vi "数据采集传输系统.vi"() -> ()   [LabVIEW 2016]
uses:
  <vilib>/Utility/miscctls.llb/LVPointTypeDef.ctl
  <vilib>/Utility/config.llb/Write Key (String).vi
  <vilib>/Utility/config.llb/Read Key (String).vi
  <vilib>/Utility/config.llb/Read Key (Boolean).vi
  <vilib>/Utility/config.llb/Read Key (I32).vi
  <vilib>/Utility/config.llb/Write Key (U32).vi
  <vilib>/Utility/config.llb/Write Key (Boolean).vi
  <vilib>/Utility/config.llb/Write Key (I32).vi
  <vilib>/Utility/config.llb/NI_LVConfig.lvlib
  data/FreeMem.dll
  <vilib>/ptbypt/NI_PtbyPt.lvlib
panel:
  in  "数组大小":i32
  in  "实时数据发送时间间隔/min":i32=1
  in  "数据组合发送":bool
  in  "日志、参数发送":bool
  in  "2011发送":bool
  in  "判断数据反馈":bool
  in  "数据发送协议":enum16{"2005-212协议", "2017-212协议"}(ring)=enum."2017-212协议"
  in  "数据发送通道":enum16{"TCP", "VISA"}(ring)
  in  "baud rate":u32=9600 caption="波特率"
  in  "VISA resource name":refnum<visa-resource-name> caption="VISA资源名称"
  in  "查询质控数据起始时间":bool
  in  "返回主界面":bool
  out "零点核查索引起始时间":string
  out "跨度核查索引起始时间":string
  out "加标回收索引起始时间":string
  out "标样核查索引起始时间":string
  out "数据接收超时指示灯":bool
  in  "重发时间":T1(ring)
  in  "重发日期":T2(ring)
  in  "锁":bool
  in  "开机启动":bool
  in  "确定更改起始时间":bool
  in  "更改起始时间":bool
  in  "数据发送起始时间":timestamp format="%<%.3X\n%Y/%m/%d>T"
  in  "每周自动重发":bool=TRUE
  in  "确定":bool
  in  "返回":bool
  in  "PW":string
  in  "MN":string
  in  "PORT":string
  in  "IP":string
  in  "站点设备":string
  in  "站点名称":string
  out "设置超时时间/min":i32=1
  out "空闲时间/s":string
  out "状态信息":T3={"1st Error to Convert "=63, "步骤 "=enum."打开连接", "元素"="实时数据", "TCP服务端掉线计数"=4, "TCP掉线时间节点"="2019/05/08 15:24:17"} {"1st Error to Convert" items=["无错误", "参数错误", "内存已满", "超出区域", "文件结束", "文件已打开", "一般文件IO错误", "未找到文件", "文件权限错误", "磁盘已满", "路径副本", "打开过多文件", "未启用", "未找到资源文件", "无法添加资源", "未找到资源", "未找到图像", "图像内存错误", "画笔不存在", "配置错误类型", "配置未找到解析段", "配置解析错误", "配置内存错误", "错误外部代码格式", "错误外部代码偏移量", "外部代码不存在", "空窗口", "销毁窗口错误", "空菜单", "打印已中止", "错误打印记录", "打印驱动程序错误", "打印时窗口错误", "打印时内存错误", "打印对话框错误", "一般打印错误", "无效设备引用句柄", "设备未找到", "设备参数错误", "设备单位错误", "无法打开设备", "设备调用已中止", "一般错误", "用户已取消", "对象ID过低", "对象ID过高", "对象不在堆中", "未知的堆", "错误DefProc ID", "DefProc不在表格中", "范围外信息", "空方法", "未知信息", "不支持管理器调用", "错误地址", "连接过程中", "连接超时", "连接过程中", "不支持网络属性", "网络错误", "正在使用的地址", "系统缺少内存", "连接已中止", "连接已拒绝", "连接未建立", "连接已建立", "连接已关闭", "初始化错误（交互应用程序管理器）", "错误事件发生", "等待无约束事件发生处理程序", "事件发生队列溢出", "错误路径", "未发出信号量", "未识别类型（交互应用程序管理器）"]}
  out "系统时间":string
  out "实时小时数据上传":bool
  out "系统状态改变":bool
  out "软件版本":string
  out "掉线指示":bool
  out "核查数据上传":bool
  out "通信状态":bool
  out "配置信息":T4
  in  "参数配置":bool
  out "查询数据发送":bool
  out "读取报文显示":string
  out "发送报文显示":string
  out "心跳包":bool
  in  "参数数值":T5={"CODMn"=TRUE, "CODCr"=TRUE, "DO"=TRUE, "铜"=TRUE, "PH"=TRUE, "氨氮"=TRUE, "比电导率"=TRUE, "水温"=TRUE, "盐度(海水)"=TRUE, "浊度"=TRUE, "总氮"=TRUE, "总磷"=TRUE, "叶绿素a"=TRUE, "藻密度"=TRUE, "水位"=TRUE, "流速"=TRUE, "瞬时流量"=TRUE, "累积流量"=TRUE}
  in  "系统编码选择框":string(combo)="地表水质量监测"
  out "主队列输出":refnum<queue>
  in  "TCP掉线时间节点":string
  out "TCP服务端掉线计数":i32
  out "元素":string
  out "步骤":T6(ring)
  out "1st Error to Convert":i32(ring)=56 items=["无错误", "参数错误", "内存已满", "超出区域", "文件结束", "文件已打开", "一般文件IO错误", "未找到文件", "文件权限错误", "磁盘已满", "路径副本", "打开过多文件", "未启用", "未找到资源文件", "无法添加资源", "未找到资源", "未找到图像", "图像内存错误", "画笔不存在", "配置错误类型", "配置未找到解析段", "配置解析错误", "配置内存错误", "错误外部代码格式", "错误外部代码偏移量", "外部代码不存在", "空窗口", "销毁窗口错误", "空菜单", "打印已中止", "错误打印记录", "打印驱动程序错误", "打印时窗口错误", "打印时内存错误", "打印对话框错误", "一般打印错误", "无效设备引用句柄", "设备未找到", "设备参数错误", "设备单位错误", "无法打开设备", "设备调用已中止", "一般错误", "用户已取消", "对象ID过低", "对象ID过高", "对象不在堆中", "未知的堆", "错误DefProc ID", "DefProc不在表格中", "范围外信息", "空方法", "未知信息", "不支持管理器调用", "错误地址", "连接过程中", "连接超时", "连接过程中", "不支持网络属性", "网络错误", "正在使用的地址", "系统缺少内存", "连接已中止", "连接已拒绝", "连接未建立", "连接已建立", "连接已关闭", "初始化错误（交互应用程序管理器）", "错误事件发生", "等待无约束事件发生处理程序", "事件发生队列溢出", "错误路径", "未发出信号量", "未识别类型（交互应用程序管理器）"]
  out "QN":string
  out "时间QN":string
  out "系统编码ST":string
  out "命令编码CN":string
  out "密码PW":string
  out "设备编码MN":string
  out "拆分包及应答Flag":string
  out "数据":string
  in  "实时数据参数选择框":T7={"水样测量数据"=FALSE, "零点核查数据"=TRUE, "跨度核查数据"=TRUE, "加标回收数据"=TRUE, "平行样数据"=FALSE, "标样核查"=TRUE, "集成干预测试"=TRUE}
  out "数据输出":string
  in  "table元素":string
  out "空闲时间":dbl
  # "数 据 采 集 传 输 系 统"
  # "读取的参数区"
  # "水样测量数据"
  # "空白测试数据"
  # "跨度核查数据"
  # "加标回收数据"
  # "平行样数据"
  # "标样核查"
  # "集成干预测试"
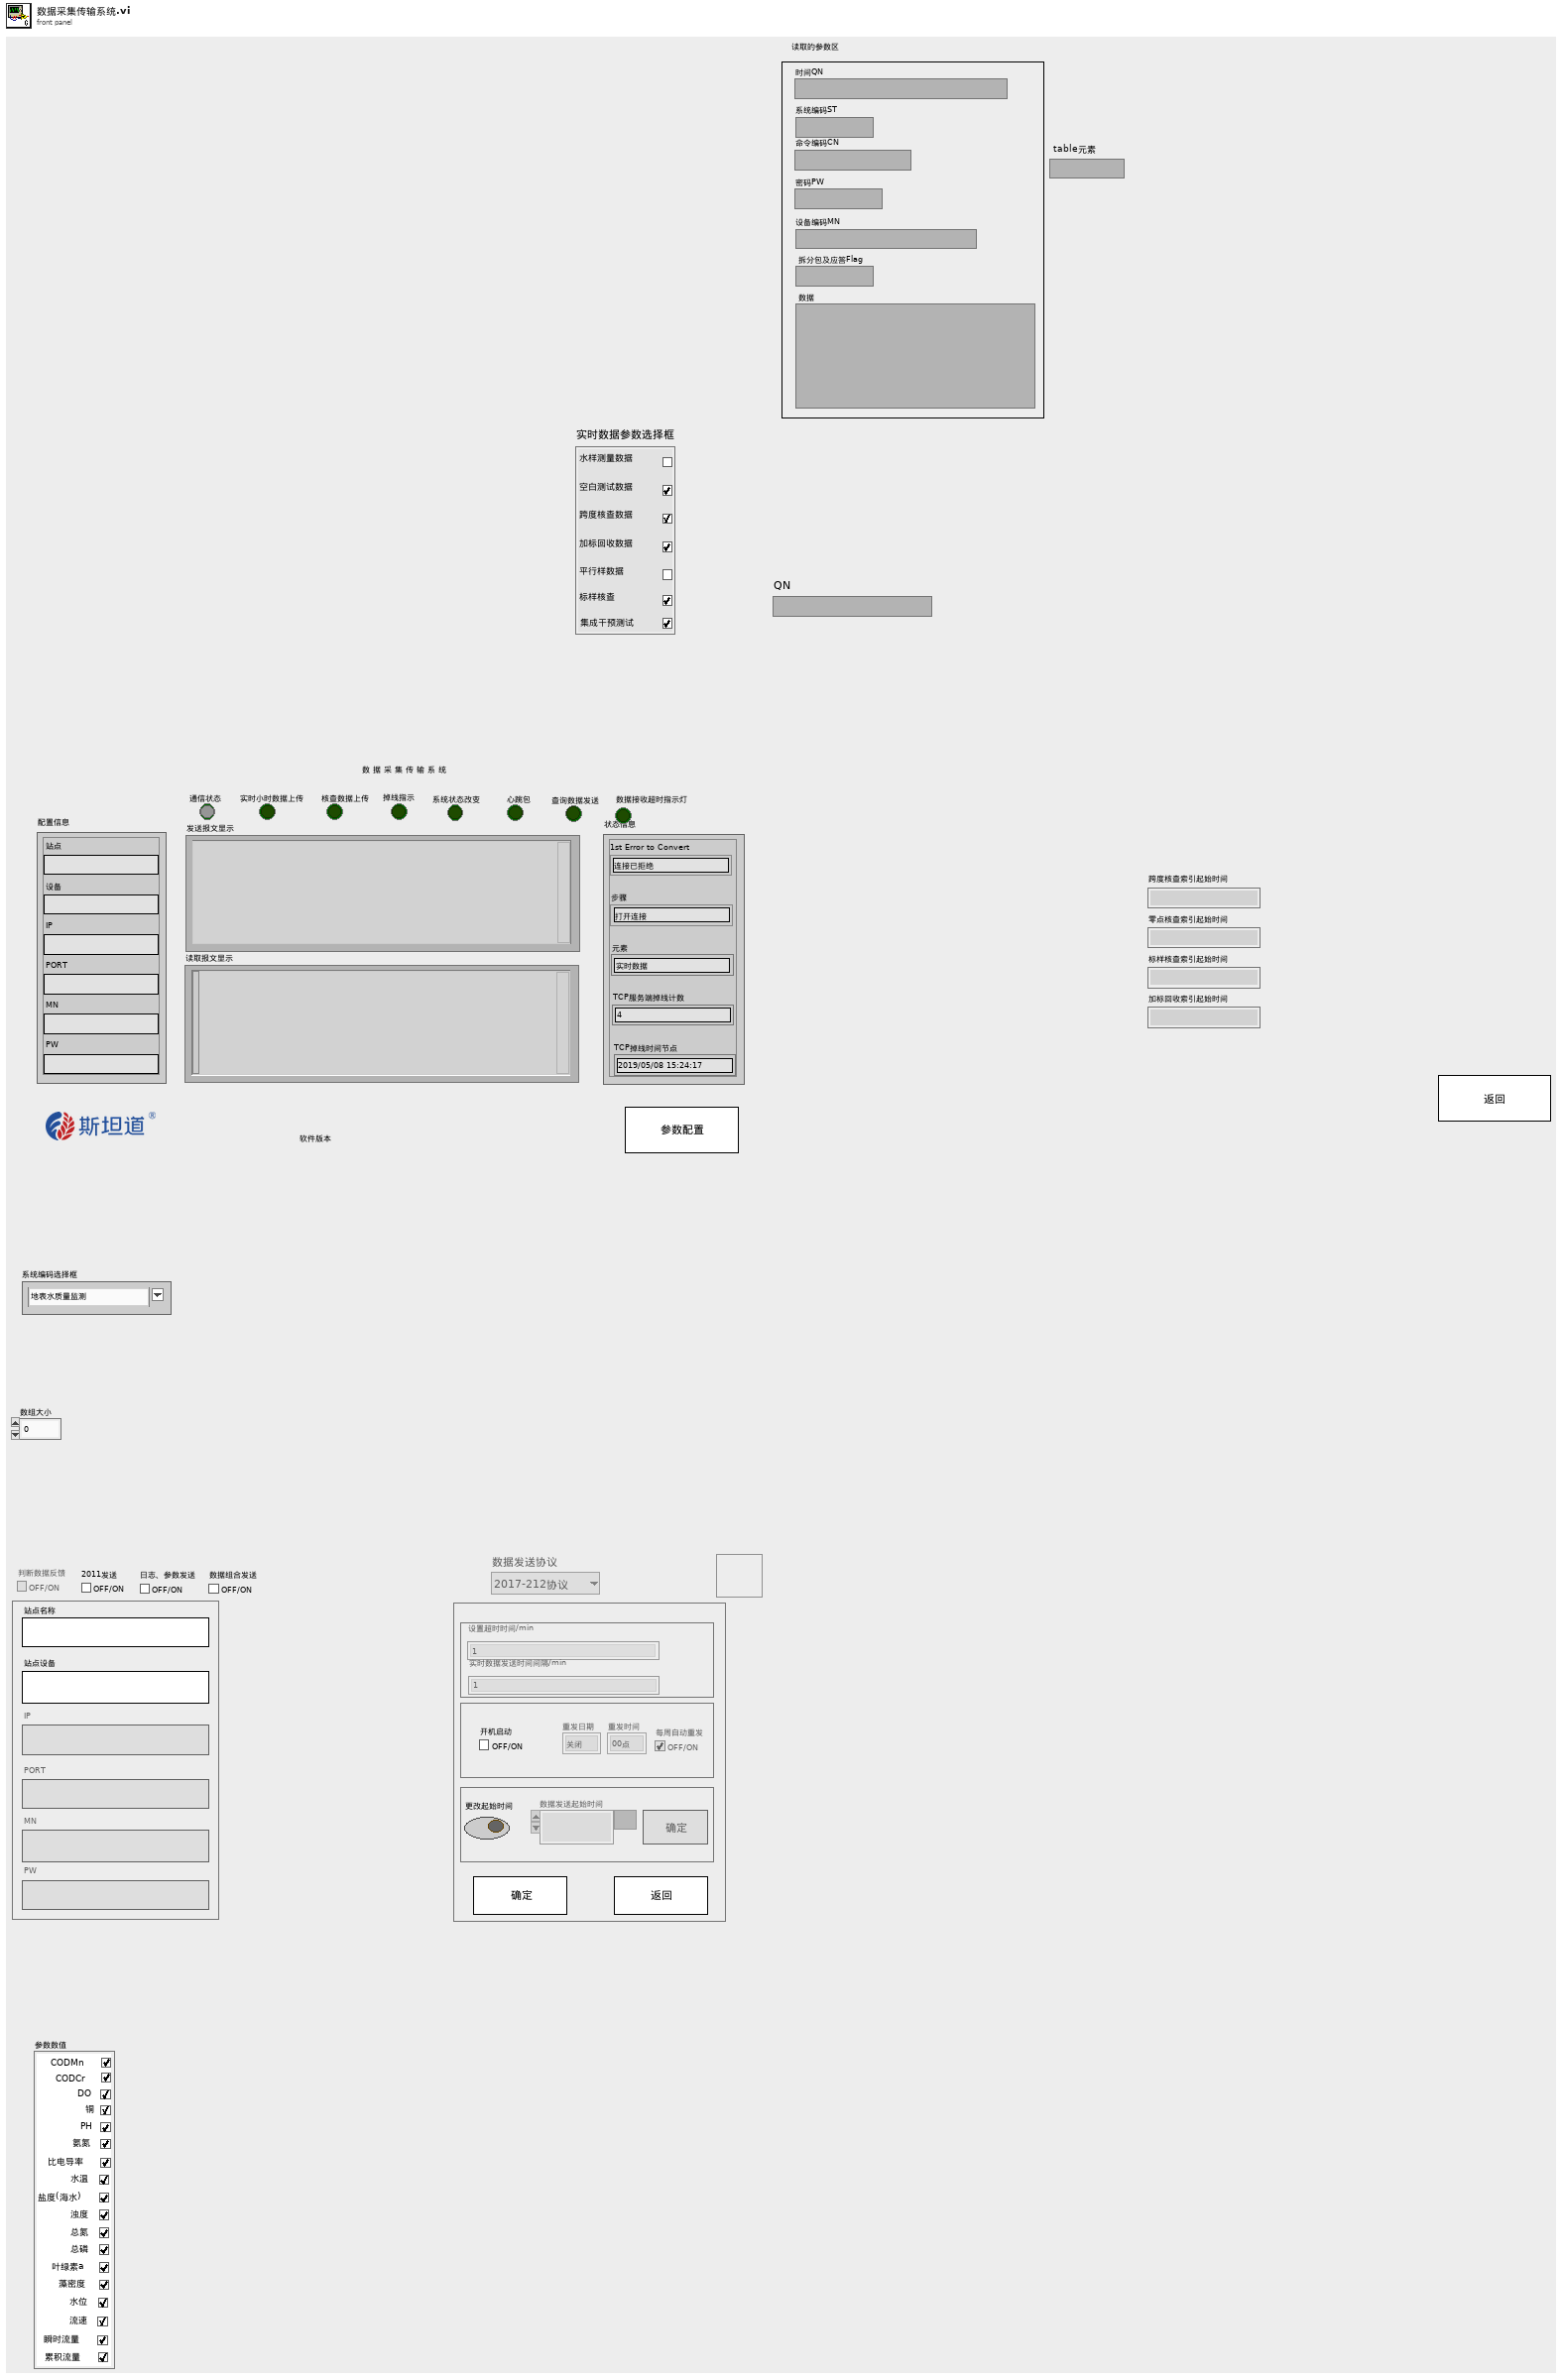
[diagram p1: front panel]
types:
  T1 = enum16{"00点", "01点", "02点", "03点", "04点", "05点", "06点", "07点", "08点", "09点", "10点", "11点", "12点", "13点", "14点", "15点", "16点", "17点", "18点", "19点", "20点", "21点", "22点", "23点"}
  T2 = enum16{"关闭", "星期日", "星期一", "星期二", "星期三", "星期四", "星期五", "星期六"}
  T3 = cluster{"1st Error to Convert ":i32, "步骤 ":enum16{"初始化", "打开连接", "表格比对", "发送数据", "读取数据", "数据处理"}, "元素":string, "TCP服务端掉线计数":i32, "TCP掉线时间节点":string}
  T4 = cluster{"站点":string, "设备":string, "IP":string, "PORT":string, "MN":string, "PW":string}
  T5 = cluster{"CODMn":bool, "CODCr":bool, "DO":bool, "铜":bool, "PH":bool, "氨氮":bool, "比电导率":bool, "水温":bool, "盐度(海水)":bool, "浊度":bool, "总氮":bool, "总磷":bool, "叶绿素a":bool, "藻密度":bool, "水位":bool, "流速":bool, "瞬时流量":bool, "累积流量":bool}
  T6 = enum16{"初始化", "打开连接", "表格比对", "发送数据", "读取数据", "数据处理"}
  T7 = cluster{"水样测量数据":bool, "零点核查数据":bool, "跨度核查数据":bool, "加标回收数据":bool, "平行样数据":bool, "标样核查":bool, "集成干预测试":bool}
  T8 = typedef "NI_LVConfig.lvlib/Config Data RefNum.ctl" = refnum<k1>
  T9 = typedef "LVDateTimeRec.ctl" = cluster{"秒数的小数部分":dbl, "秒":i32, "分":i32, "时":i32, "日":i32, "月":i32, "年":i32, "天数（周）":i32, "天数（年）":i32, "DST":i32}
  T10 = enum8{"Enabled", "Disabled", "Disabled and Grayed Out"}
  T11 = typedef "LVPointTypeDef.ctl" = cluster{"Horizontal":i16, "Vertical":i16}
  T12 = enum16{"水样测试", "小时数据", "日志信息", "报警信息", "零点核查", "标样核查", "平行样", "加标回收"}
  T13 = typedef "imagedata.ctl" = cluster{"image type":i32, "image depth":i32, "image":u8[], "mask":u8[], "colors":u32[], "Rectangle":cluster{"left":i16, "top":i16, "right":i16, "bottom":i16}}
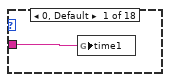
[diagram p5: hidden frame]
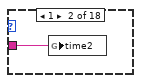
[diagram p6: hidden frame]
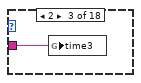
[diagram p7: hidden frame]
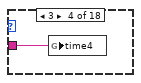
[diagram p8: hidden frame]
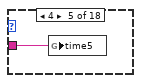
[diagram p9: hidden frame]
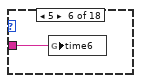
[diagram p10: hidden frame]
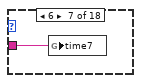
[diagram p11: hidden frame]
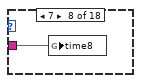
[diagram p12: hidden frame]
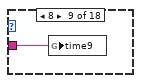
[diagram p13: hidden frame]
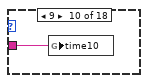
[diagram p14: hidden frame]
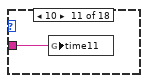
[diagram p15: hidden frame]
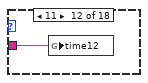
[diagram p16: hidden frame]
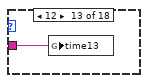
[diagram p17: hidden frame]
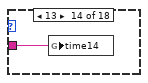
[diagram p18: hidden frame]
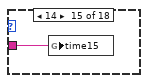
[diagram p19: hidden frame]
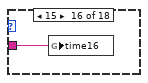
[diagram p20: hidden frame]
diagram:
  w37 = 0 ("索引")
  # "上传本地时间点的实时数据"
  # "目前时间太短，如果掉线了，数据存不了临时表格"
  n1 = Cluster To Array(cluster="参数数值") -> (array=w47:bool[])
  n2 = for {
    tunnel: w47 -> [_] mode=indexing
    tunnel: [w73] -> _
    i -> [w73]
    w62 = "线程一数据重发功能" ("section")
    # "初始化水样搜索起始时间"
    n3 = case shown="3" w73 {
      tunnel: [w104 w106 w108 w110 w112 w114 w116 w118 w120 w122 w124 w126 w128 w130 w132 w134 w136 w138] -> w77
      frame 0, Default {
        n4 = control-ref of="CODMn"() -> (w105:refnum<vi>)
        n5 = property class="Bool (严格)"(reference=w105) -> ("Label.Text"=w104:string)  [unwired: 1 in, 2 out]
      }
      frame 1 {
        n6 = control-ref of="CODCr"() -> (w107:refnum<vi>)
        n7 = property class="Bool (严格)"(reference=w107) -> ("Label.Text"=w106:string)  [unwired: 1 in, 2 out]
      }
      frame 2 {
        n8 = control-ref of="DO"() -> (w109:refnum<vi>)
        n9 = property class="Bool (严格)"(reference=w109) -> ("Label.Text"=w108:string)  [unwired: 1 in, 2 out]
      }
      frame 3 {
        n10 = control-ref of="铜"() -> (w111:refnum<vi>)
        n11 = property class="Bool (严格)"(reference=w111) -> ("Label.Text"=w110:string)  [unwired: 1 in, 2 out]
      }
      frame 4 {
        n12 = control-ref of="PH"() -> (w113:refnum<vi>)
        n13 = property class="Bool (严格)"(reference=w113) -> ("Label.Text"=w112:string)  [unwired: 1 in, 2 out]
      }
      frame 5 {
        n14 = control-ref of="氨氮"() -> (w115:refnum<vi>)
        n15 = property class="Bool (严格)"(reference=w115) -> ("Label.Text"=w114:string)  [unwired: 1 in, 2 out]
      }
      frame 6 {
        n16 = control-ref of="比电导率"() -> (w117:refnum<vi>)
        n17 = property class="Bool (严格)"(reference=w117) -> ("Label.Text"=w116:string)  [unwired: 1 in, 2 out]
      }
      frame 7 {
        n18 = control-ref of="水温"() -> (w119:refnum<vi>)
        n19 = property class="Bool (严格)"(reference=w119) -> ("Label.Text"=w118:string)  [unwired: 1 in, 2 out]
      }
      frame 8 {
        n20 = control-ref of="盐度(海水)"() -> (w121:refnum<vi>)
        n21 = property class="Bool (严格)"(reference=w121) -> ("Label.Text"=w120:string)  [unwired: 1 in, 2 out]
      }
      frame 9 {
        n22 = control-ref of="浊度"() -> (w123:refnum<vi>)
        n23 = property class="Bool (严格)"(reference=w123) -> ("Label.Text"=w122:string)  [unwired: 1 in, 2 out]
      }
      frame 10 {
        n24 = control-ref of="总氮"() -> (w125:refnum<vi>)
        n25 = property class="Bool (严格)"(reference=w125) -> ("Label.Text"=w124:string)  [unwired: 1 in, 2 out]
      }
      frame 11 {
        n26 = control-ref of="总磷"() -> (w127:refnum<vi>)
        n27 = property class="Bool (严格)"(reference=w127) -> ("Label.Text"=w126:string)  [unwired: 1 in, 2 out]
      }
      frame 12 {
        n28 = control-ref of="叶绿素a"() -> (w129:refnum<vi>)
        n29 = property class="Bool (严格)"(reference=w129) -> ("Label.Text"=w128:string)  [unwired: 1 in, 2 out]
      }
      frame 13 {
        n30 = control-ref of="藻密度"() -> (w131:refnum<vi>)
        n31 = property class="Bool (严格)"(reference=w131) -> ("Label.Text"=w130:string)  [unwired: 1 in, 2 out]
      }
      frame 14 {
        n32 = control-ref of="水位"() -> (w133:refnum<vi>)
        n33 = property class="Bool (严格)"(reference=w133) -> ("Label.Text"=w132:string)  [unwired: 1 in, 2 out]
      }
      frame 15 {
        n34 = control-ref of="流速"() -> (w135:refnum<vi>)
        n35 = property class="Bool (严格)"(reference=w135) -> ("Label.Text"=w134:string)  [unwired: 1 in, 2 out]
      }
      frame 16 {
        n36 = control-ref of="瞬时流量"() -> (w137:refnum<vi>)
        n37 = property class="Bool (严格)"(reference=w137) -> ("Label.Text"=w136:string)  [unwired: 1 in, 2 out]
      }
      frame 17 {
        n38 = control-ref of="累积流量"() -> (w139:refnum<vi>)
        n39 = property class="Bool (严格)"(reference=w139) -> ("Label.Text"=w138:string)  [unwired: 1 in, 2 out]
      }
    }
    n40 = call <vilib>:"Application Directory.vi"() -> ("Application Directory"=w83:path)
    n41 = Build Path(base path=w83, name or relative path="data\\Set.ini" ("名称或相对路径")) -> (appended path=w81:path)
    n42 = call <vilib>:"Open Config Data.vi"("configuration file path"=w81) -> ("error out"=w79:errorcluster, "refnum"=w80:T8)  [unwired: 8 in, 1 out]
    n43 = call-poly <vilib>:"Read Key.vi"("section"="线程一数据搜索起始时间", "error in (no error)"=w79, "key"=w77, "refnum"=w80) -> ("error out"=w71:errorcluster, "value"=w74:string, "refnum out"=w72:T8)  [unwired: 4 in, 1 out]
    n44 = Empty String/Path?(string/path=w74) -> (empty?=w76:bool)
    n45 = case shown="真" w76 {
      tunnel: [w84 "1904/01/01 00:00:00"] -> w75
      tunnel: w74 -> [w84 _]
      frame False {
      }
      frame True {
      }
    }
    n46 = call-poly <vilib>:"Read Key.vi"("section"=w62, "error in (no error)"=w71, "key"="重发功能", "refnum"=w72) -> ("error out"=w65:errorcluster, "value"=w69:bool, "refnum out"=w66:T8)  [unwired: 4 in, 1 out]
    n47 = local write "每周自动重发"(w69) -> ()
    n48 = call-poly <vilib>:"Read Key.vi"("section"=w62, "error in (no error)"=w65, "key"="重发日期", "refnum"=w66) -> ("error out"=w63:errorcluster, "value"=w59:i32, "refnum out"=w64:T8)  [unwired: 4 in, 1 out]
    n49 = local write "重发日期"(w59) -> ()
    n50 = case shown="3" w73 {
      tunnel: w75 -> [w86 w87 w88 w89 w90 w91 w92 w93 w94 w95 w96 w97 w98 w99 w100 w101 w102 w103]
      frame 0, Default {
        n51 = global write "全局 水样时间.vi" "time1"(w86) -> ()
      }
      frame 1 {
        n52 = global write "全局 水样时间.vi" "time2"(w87) -> ()
      }
      frame 2 {
        n53 = global write "全局 水样时间.vi" "time3"(w88) -> ()
      }
      frame 3 {
        n54 = global write "全局 水样时间.vi" "time4"(w89) -> ()
      }
      frame 4 {
        n55 = global write "全局 水样时间.vi" "time5"(w90) -> ()
      }
      frame 5 {
        n56 = global write "全局 水样时间.vi" "time6"(w91) -> ()
      }
      frame 6 {
        n57 = global write "全局 水样时间.vi" "time7"(w92) -> ()
      }
      frame 7 {
        n58 = global write "全局 水样时间.vi" "time8"(w93) -> ()
      }
      frame 8 {
        n59 = global write "全局 水样时间.vi" "time9"(w94) -> ()
      }
      frame 9 {
        n60 = global write "全局 水样时间.vi" "time10"(w95) -> ()
      }
      frame 10 {
        n61 = global write "全局 水样时间.vi" "time11"(w96) -> ()
      }
      frame 11 {
        n62 = global write "全局 水样时间.vi" "time12"(w97) -> ()
      }
      frame 12 {
        n63 = global write "全局 水样时间.vi" "time13"(w98) -> ()
      }
      frame 13 {
        n64 = global write "全局 水样时间.vi" "time14"(w99) -> ()
      }
      frame 14 {
        n65 = global write "全局 水样时间.vi" "time15"(w100) -> ()
      }
      frame 15 {
        n66 = global write "全局 水样时间.vi" "time16"(w101) -> ()
      }
      frame 16 {
        n67 = global write "全局 水样时间.vi" "time17"(w102) -> ()
      }
      frame 17 {
        n68 = global write "全局 水样时间.vi" "time18"(w103) -> ()
      }
    }
    n69 = call-poly <vilib>:"Read Key.vi"("section"=w62, "error in (no error)"=w63, "key"="重发时间", "refnum"=w64) -> ("error out"=w60:errorcluster, "value"=w58:i32, "refnum out"=w61:T8)  [unwired: 4 in, 1 out]
    n70 = local write "重发时间"(w58) -> ()
    n71 = call <vilib>:"Close Config Data.vi"("error in (no error)"=w60, "refnum"=w61) -> ()  [unwired: 8 in, 2 out]
  }
  n72 = vi-ref "数据传输系统.lvlib:核查数据和日志信息入发送队列 (子VI).vi"() -> (w20:refnum<vi>)
  n73 = vi-ref "数据传输系统.lvlib:主动上传工控机周期和模式 (子VI).vi"() -> (w29:refnum<vi>)
  n74 = vi-ref "数据传输系统.lvlib:核查数据和日志信息出发送队列 (子VI).vi"() -> (w11:refnum<vi>)
  n75 = local read "实时小时数据上传"() -> (w16:bool)
  n76 = property class="VI"(reference=w29) -> ("Name"=w30:string)  [unwired: 1 in, 2 out]
  n77 = property class="VI"(reference=w11) -> ("Name"=w10:string)  [unwired: 1 in, 2 out]
  n78 = local read "查询数据发送"() -> (w3:bool)
  n79 = local read "核查数据上传"() -> (w19:bool)
  n80 = local read "查询数据发送"() -> (w18:bool)
  n81 = local read "日志、参数发送"() -> (w14:bool)
  n82 = property class="VI"(reference=w20) -> ("Name"=w27:string)  [unwired: 1 in, 2 out]
  n83 = local read "步骤"() -> (w17:T6)
  n84 = local read "数据发送协议"() -> (w15:enum16{"2005-212协议", "2017-212协议"})
  n85 = Open VI Reference(type specifier VI Refnum (for type only)=refnum<vi> refnum, vi path=w30, options=128 ("选项")) -> (vi reference=w32:refnum<vi>, error out=w34:errorcluster)  [unwired: 3 in]
  n86 = Open VI Reference(type specifier VI Refnum (for type only)=refnum<vi> refnum, vi path=w10, options=128 ("选项")) -> (vi reference=w8:refnum<vi>, error out=w6:errorcluster)  [unwired: 3 in]
  n87 = Open VI Reference(type specifier VI Refnum (for type only)=refnum<vi> refnum, vi path=w27, options=128 ("选项")) -> (vi reference=w25:refnum<vi>, error out=w23:errorcluster)  [unwired: 3 in]
  n88 = call-by-ref "?"(reference=w32, error in=w34) -> (reference out=w36:refnum<vi>, error out=w35:errorcluster, "系统状态改变"=→"系统状态改变":bool)  [unwired: 11 in]
  n89 = call-by-ref "?"(reference=w8, error in=w6, "查询数据发送"=w3) -> (reference out=w4:refnum<vi>, error out=w5:errorcluster, "核查数据上传"=→"核查数据上传":bool)  [unwired: 10 in]
  n90 = call-by-ref "?"(reference=w25, error in=w23, "实时数据参数选择框"="实时数据参数选择框", "实时数据发送时间间隔/min"="实时数据发送时间间隔/min", "日志、参数发送输入"=w14, "数据发送协议输入"=w15, "实时小时数据上传输入"=w16, "步骤输入"=w17, "查询数据发送输入"=w18, "核查数据上传输入"=w19) -> (reference out=w21:refnum<vi>, error out=w22:errorcluster)  [unwired: 4 in]
  n91 = Close Reference(reference=w36, error in (no error)=w35) -> ()  [unwired: 1 out]
  n92 = Close Reference(reference=w4, error in (no error)=w5) -> ()  [unwired: 1 out]
  n93 = Close Reference(reference=w21, error in (no error)=w22) -> ()  [unwired: 1 out]
  n94 = while "While循环" {
    tunnel: [w154] -> _
    stop <- FALSE stop-if-true
    w145 = FALSE ("小时数据上传")
    # "2017，2005版协议实时、小时数据出数据就单参数上传"
    n95 = local read "查询数据发送"() -> (w147:bool)
    n96 = local read "核查数据上传"() -> (w146:bool)
    n97 = global read "全局 数据发送重叠.vi" "掉线指示灯"() -> (w141:bool)
    n98 = local read "步骤"() -> (w153:T6)
    n99 = local write "实时小时数据上传"(w145) -> ()
    n100 = global write "全局 数据发送重叠.vi" "主动上报数据中"(w145) -> ()
    n101 = Greater Or Equal?(x="数组大小", y=17) -> (x >= y?=w150:bool)
    n102 = Not(x=w141) -> (.not. x?=w140:bool)
    n103 = Not(x=w147) -> (.not. x?=w144:bool)
    n104 = Not(x=w146) -> (.not. x?=w143:bool)
    n105 = Equal?(x=w153, y=T6."读取数据" ("步骤")) -> (x = y?=w151:bool)
    n106 = Wait (ms)(milliseconds to wait=u32 75430 ("等待时间（毫秒）")) -> ()  [unwired: 1 out]
    n107 = Compound Arithmetic op=AND ("复合运算")(w151, w140, w150, w144, w143) -> (w148:bool)
    n108 = case shown="真" w148 {
      tunnel: [_ w159] -> w154
      frame False {
        w157 = FALSE ("小时数据上传")
        n109 = local write "实时小时数据上传"(w157) -> ()
        n110 = global write "全局 数据发送重叠.vi" "主动上报数据中"(w157) -> ()
      }
      frame True {
        n111 = global read "断电保存全局.vi" "数据组合发送"() -> (w158:bool)
        n112 = case shown="假" w158 {
          tunnel: [w160 _] -> w159
          frame False {
            # "数据非整点触发，而是实时触发，分条发送"
            n113 = flat-sequence {
              tunnel: [w164] -> w161
              tunnel: [w445] -> w160
              tunnel: w161 -> [w445]
              frame #0 {
                w163 = TRUE ("小时数据上传")
                n114 = global read "断电保存全局.vi" "数据发送协议"() -> (w162:enum16{"2005-212协议", "2017-212协议"})
                n115 = global write "全局 数据发送重叠.vi" "主动上报数据中"(w163) -> ()
                n116 = case shown="\"2017-212协议\", 默认" w162 {
                  tunnel: [_ w266] -> w164
                  frame "2005-212协议" {
                    n117 = local read "参数数值"() -> (w165:T5)
                    n118 = Cluster To Array(cluster=w165) -> (array=w168:bool[])
                    n119 = for {
                      tunnel: w168 -> [_] mode=indexing
                      tunnel: [w211] -> w167
                      i -> [w209]
                      (unwired) " where 时间 between #"
                      w207 = "database1.mdb" ("database")
                      (unwired) "'and 数据类型 ='N' and 时间 between "
                      n120 = case shown="12" w209 {
                        tunnel: [w230 w232 w234 w236 w238 w240 w242 w244 w246 w248 w250 w252 w254 w256 w258 w260 w262 w264] -> w208
                        frame 0, Default {
                          n121 = control-ref of="CODMn"() -> (w231:refnum<vi>)
                          n122 = property class="Bool (严格)"(reference=w231) -> ("Label.Text"=w230:string)  [unwired: 1 in, 2 out]
                        }
                        frame 1 {
                          n123 = control-ref of="CODCr"() -> (w233:refnum<vi>)
                          n124 = property class="Bool (严格)"(reference=w233) -> ("Label.Text"=w232:string)  [unwired: 1 in, 2 out]
                        }
                        frame 2 {
                          n125 = control-ref of="DO"() -> (w235:refnum<vi>)
                          n126 = property class="Bool (严格)"(reference=w235) -> ("Label.Text"=w234:string)  [unwired: 1 in, 2 out]
                        }
                        frame 3 {
                          n127 = control-ref of="铜"() -> (w237:refnum<vi>)
                          n128 = property class="Bool (严格)"(reference=w237) -> ("Label.Text"=w236:string)  [unwired: 1 in, 2 out]
                        }
                        frame 4 {
                          n129 = control-ref of="PH"() -> (w239:refnum<vi>)
                          n130 = property class="Bool (严格)"(reference=w239) -> ("Label.Text"=w238:string)  [unwired: 1 in, 2 out]
                        }
                        frame 5 {
                          n131 = control-ref of="氨氮"() -> (w241:refnum<vi>)
                          n132 = property class="Bool (严格)"(reference=w241) -> ("Label.Text"=w240:string)  [unwired: 1 in, 2 out]
                        }
                        frame 6 {
                          n133 = control-ref of="比电导率"() -> (w243:refnum<vi>)
                          n134 = property class="Bool (严格)"(reference=w243) -> ("Label.Text"=w242:string)  [unwired: 1 in, 2 out]
                        }
                        frame 7 {
                          n135 = control-ref of="水温"() -> (w245:refnum<vi>)
                          n136 = property class="Bool (严格)"(reference=w245) -> ("Label.Text"=w244:string)  [unwired: 1 in, 2 out]
                        }
                        frame 8 {
                          n137 = control-ref of="盐度(海水)"() -> (w247:refnum<vi>)
                          n138 = property class="Bool (严格)"(reference=w247) -> ("Label.Text"=w246:string)  [unwired: 1 in, 2 out]
                        }
                        frame 9 {
                          n139 = control-ref of="浊度"() -> (w249:refnum<vi>)
                          n140 = property class="Bool (严格)"(reference=w249) -> ("Label.Text"=w248:string)  [unwired: 1 in, 2 out]
                        }
                        frame 10 {
                          n141 = control-ref of="总氮"() -> (w251:refnum<vi>)
                          n142 = property class="Bool (严格)"(reference=w251) -> ("Label.Text"=w250:string)  [unwired: 1 in, 2 out]
                        }
                        frame 11 {
                          n143 = control-ref of="总磷"() -> (w253:refnum<vi>)
                          n144 = property class="Bool (严格)"(reference=w253) -> ("Label.Text"=w252:string)  [unwired: 1 in, 2 out]
                        }
                        frame 12 {
                          n145 = control-ref of="叶绿素a"() -> (w255:refnum<vi>)
                          n146 = property class="Bool (严格)"(reference=w255) -> ("Label.Text"=w254:string)  [unwired: 1 in, 2 out]
                        }
                        frame 13 {
                          n147 = control-ref of="藻密度"() -> (w257:refnum<vi>)
                          n148 = property class="Bool (严格)"(reference=w257) -> ("Label.Text"=w256:string)  [unwired: 1 in, 2 out]
                        }
                        frame 14 {
                          n149 = control-ref of="水位"() -> (w259:refnum<vi>)
                          n150 = property class="Bool (严格)"(reference=w259) -> ("Label.Text"=w258:string)  [unwired: 1 in, 2 out]
                        }
                        frame 15 {
                          n151 = control-ref of="流速"() -> (w261:refnum<vi>)
                          n152 = property class="Bool (严格)"(reference=w261) -> ("Label.Text"=w260:string)  [unwired: 1 in, 2 out]
                        }
                        frame 16 {
                          n153 = control-ref of="瞬时流量"() -> (w263:refnum<vi>)
                          n154 = property class="Bool (严格)"(reference=w263) -> ("Label.Text"=w262:string)  [unwired: 1 in, 2 out]
                        }
                        frame 17 {
                          n155 = control-ref of="累积流量"() -> (w265:refnum<vi>)
                          n156 = property class="Bool (严格)"(reference=w265) -> ("Label.Text"=w264:string)  [unwired: 1 in, 2 out]
                        }
                      }
                      n157 = global read "断电保存全局.vi" "数据发送协议"() -> (w205:enum16{"2005-212协议", "2017-212协议"})
                      n158 = call "主动发送数据生成Condition(子VI).vi"("数据发送协议"=w205, "database"=w207, "Label.Text"=w208, "数值"=w209) -> ("CONDITION"=w206:string)  [unwired: 7 in]
                      n159 = call "SQL查询.vi"("condition"=w206, "table输入"=w208, "database"=w207) -> ("error out"=w211:errorcluster, "data"=w210:string[][])  [unwired: 7 in]
                      n160 = case shown="3" w209 {
                        tunnel: w210 -> [w212 w213 w214 w215 w216 w217 w218 w219 w220 w221 w222 w223 w224 w225 w226 w227 w228 w229]
                        frame 0, Default {
                          n161 = global write "全局 所有参数.vi" "CODMn"(w212) -> ()
                        }
                        frame 1 {
                          n162 = global write "全局 所有参数.vi" "CODCr"(w213) -> ()
                        }
                        frame 2 {
                          n163 = global write "全局 所有参数.vi" "DO"(w214) -> ()
                        }
                        frame 3 {
                          n164 = global write "全局 所有参数.vi" "铜"(w215) -> ()
                        }
                        frame 4 {
                          n165 = global write "全局 所有参数.vi" "PH"(w216) -> ()
                        }
                        frame 5 {
                          n166 = global write "全局 所有参数.vi" "氨氮"(w217) -> ()
                        }
                        frame 6 {
                          n167 = global write "全局 所有参数.vi" "电导率"(w218) -> ()
                        }
                        frame 7 {
                          n168 = global write "全局 所有参数.vi" "水温"(w219) -> ()
                        }
                        frame 8 {
                          n169 = global write "全局 所有参数.vi" "盐度"(w220) -> ()
                        }
                        frame 9 {
                          n170 = global write "全局 所有参数.vi" "浊度"(w221) -> ()
                        }
                        frame 10 {
                          n171 = global write "全局 所有参数.vi" "总氮"(w222) -> ()
                        }
                        frame 11 {
                          n172 = global write "全局 所有参数.vi" "总磷"(w223) -> ()
                        }
                        frame 12 {
                          n173 = global write "全局 所有参数.vi" "叶绿素"(w224) -> ()
                        }
                        frame 13 {
                          n174 = global write "全局 所有参数.vi" "藻密度"(w225) -> ()
                        }
                        frame 14 {
                          n175 = global write "全局 所有参数.vi" "水位"(w226) -> ()
                        }
                        frame 15 {
                          n176 = global write "全局 所有参数.vi" "流速"(w227) -> ()
                        }
                        frame 16 {
                          n177 = global write "全局 所有参数.vi" "瞬时流量"(w228) -> ()
                        }
                        frame 17 {
                          n178 = global write "全局 所有参数.vi" "累积流量"(w229) -> ()
                        }
                      }
                    }
                    n179 = flat-sequence {
                      tunnel: w167 -> [w169]
                      tunnel: [w169] -> w166
                      tunnel: w166 -> [w175]
                      tunnel: [w174] -> _
                      frame #0 {
                        n180 = global write "全局 小时数据发送次数.vi" "小时数据发送次数"(0 ("小时数据发送次数")) -> ()
                        n181 = call "数据处理直接插入整合 (子VI).vi"() -> ()  [unwired: 12 in]
                        n182 = global write "全局1.vi" "枚举"(enum16{"返回请求应答", "上传数据", "返回执行结果"}."上传数据" ("枚举")) -> ()
                        n183 = global write "全局 实时数据参数.vi" "实时数据参数"("水样测试" ("实时数据参数")) -> ()
                        n184 = global write "全局 水样时间.vi" "选择发送的参数"("氨氮" ("选择发送的参数")) -> ()
                      }
                      frame #1 {
                        # "实时数据的大小"
                        n185 = flat-sequence {
                          tunnel: [w183] -> w178
                          tunnel: [w185] -> w176
                          tunnel: w175 -> [w184]
                          tunnel: w178 -> [_]
                          tunnel: [w194] -> w177
                          tunnel: w176 -> [w194]
                          tunnel: w177 -> [w202]
                          tunnel: [w196] -> w174
                          frame #0 {
                            n186 = Get Date/Time In Seconds() -> (seconds since 1Jan1904=w189:timestamp)
                            n187 = Format Date/Time String(time format string (%c)="%Y%m%d%H%M%S%3u" ("时间格式字符串(%c)"), seconds (now)=w189) -> (date/time string=w190:string)  [unwired: 1 in]
                            n188 = Search and Replace String(input string=w190, search string="." ("搜索字符串")) -> (result string=w192:string)  [unwired: 6 in, 3 out]
                            n189 = global read "断电保存全局.vi" "MN"() -> (w181:string)
                            n190 = global read "断电保存全局.vi" "PW"() -> (w180:string)
                            n191 = call "数据编码.vi"("table输入"="小时数据" ("新元素/子数组"), "QN"=w192, "MN"=w181, "PW"=w180) -> ("错误常量"=w179:errorcluster, "通讯包字符串"=w183:string)  [unwired: 10 in]
                            n192 = Build Array(w183) -> (w186:string[])
                            n193 = global write "全局1.vi" "发送报文显示"(w183) -> ()
                            n194 = call "发送数据记录到文档(子VI).vi"("错误输入"=w184, "数组"=w186) -> ("错误输出"=w185:errorcluster)  [unwired: 8 in]
                            n195 = call "通信状态入队列.vi"("错误输入（无错误）"=w179, "枚举"=enum16{"打开连接", "发送数据", "读取数据", "数据处理", "关闭连接"}."发送数据") -> ()  [unwired: 9 in, 1 out]
                          }
                          frame #1 {
                            n196 = global write "全局 小时数据发送次数.vi" "小时数据发送次数"(0 ("小时数据发送次数")) -> ()
                            n197 = Wait (ms)(milliseconds to wait=u32 500 ("等待时间（毫秒）")) -> ()  [unwired: 1 out]
                          }
                          frame #2 {
                            n198 = global read "断电保存全局.vi" "MN"() -> (w198:string)
                            n199 = global read "断电保存全局.vi" "PW"() -> (w199:string)
                            n200 = call "数据编码.vi"("table输入"="实时数据" ("新元素/子数组"), "错误常量 2"=w202, "MN"=w198, "PW"=w199) -> ("错误常量"=w197:errorcluster, "通讯包字符串"=w201:string)  [unwired: 10 in]
                            n201 = Build Array(w201) -> (w204:string[])
                            n202 = global write "全局1.vi" "发送报文显示"(w201) -> ()
                            n203 = call "发送数据记录到文档(子VI).vi"("数组"=w204) -> ()  [unwired: 9 in, 1 out]
                            n204 = call "通信状态入队列.vi"("错误输入（无错误）"=w197, "枚举"=enum16{"打开连接", "发送数据", "读取数据", "数据处理", "关闭连接"}."发送数据") -> ("错误输出"=w196:errorcluster)  [unwired: 9 in]
                          }
                        }
                      }
                    }
                  }
                  frame "2017-212协议", Default {
                    n205 = local read "参数数值"() -> (w268:T5)
                    n206 = Cluster To Array(cluster=w268) -> (array=w267:bool[])
                    n207 = for {
                      tunnel: w267 -> [_] mode=indexing
                      tunnel: [w273] -> w266 mode=indexing
                      tunnel: [w273] -> _
                      i -> [w272]
                      (unwired) " where 时间 between #"
                      w271 = "database1.mdb" ("database")
                      (unwired) "'and 数据类型 ='N' and 时间 between "
                      w287 = 0 ("索引 (行)")
                      n208 = case shown="3" w272 {
                        tunnel: [w408 w410 w412 w414 w416 w418 w420 w422 w424 w426 w428 w430 w432 w434 w436 w438 w440 w442] -> w270
                        frame 0, Default {
                          n209 = control-ref of="CODMn"() -> (w409:refnum<vi>)
                          n210 = property class="Bool (严格)"(reference=w409) -> ("Label.Text"=w408:string)  [unwired: 1 in, 2 out]
                        }
                        frame 1 {
                          n211 = control-ref of="CODCr"() -> (w411:refnum<vi>)
                          n212 = property class="Bool (严格)"(reference=w411) -> ("Label.Text"=w410:string)  [unwired: 1 in, 2 out]
                        }
                        frame 2 {
                          n213 = control-ref of="DO"() -> (w413:refnum<vi>)
                          n214 = property class="Bool (严格)"(reference=w413) -> ("Label.Text"=w412:string)  [unwired: 1 in, 2 out]
                        }
                        frame 3 {
                          n215 = control-ref of="铜"() -> (w415:refnum<vi>)
                          n216 = property class="Bool (严格)"(reference=w415) -> ("Label.Text"=w414:string)  [unwired: 1 in, 2 out]
                        }
                        frame 4 {
                          n217 = control-ref of="PH"() -> (w417:refnum<vi>)
                          n218 = property class="Bool (严格)"(reference=w417) -> ("Label.Text"=w416:string)  [unwired: 1 in, 2 out]
                        }
                        frame 5 {
                          n219 = control-ref of="氨氮"() -> (w419:refnum<vi>)
                          n220 = property class="Bool (严格)"(reference=w419) -> ("Label.Text"=w418:string)  [unwired: 1 in, 2 out]
                        }
                        frame 6 {
                          n221 = control-ref of="比电导率"() -> (w421:refnum<vi>)
                          n222 = property class="Bool (严格)"(reference=w421) -> ("Label.Text"=w420:string)  [unwired: 1 in, 2 out]
                        }
                        frame 7 {
                          n223 = control-ref of="水温"() -> (w423:refnum<vi>)
                          n224 = property class="Bool (严格)"(reference=w423) -> ("Label.Text"=w422:string)  [unwired: 1 in, 2 out]
                        }
                        frame 8 {
                          n225 = control-ref of="盐度(海水)"() -> (w425:refnum<vi>)
                          n226 = property class="Bool (严格)"(reference=w425) -> ("Label.Text"=w424:string)  [unwired: 1 in, 2 out]
                        }
                        frame 9 {
                          n227 = control-ref of="浊度"() -> (w427:refnum<vi>)
                          n228 = property class="Bool (严格)"(reference=w427) -> ("Label.Text"=w426:string)  [unwired: 1 in, 2 out]
                        }
                        frame 10 {
                          n229 = control-ref of="总氮"() -> (w429:refnum<vi>)
                          n230 = property class="Bool (严格)"(reference=w429) -> ("Label.Text"=w428:string)  [unwired: 1 in, 2 out]
                        }
                        frame 11 {
                          n231 = control-ref of="总磷"() -> (w431:refnum<vi>)
                          n232 = property class="Bool (严格)"(reference=w431) -> ("Label.Text"=w430:string)  [unwired: 1 in, 2 out]
                        }
                        frame 12 {
                          n233 = control-ref of="叶绿素a"() -> (w433:refnum<vi>)
                          n234 = property class="Bool (严格)"(reference=w433) -> ("Label.Text"=w432:string)  [unwired: 1 in, 2 out]
                        }
                        frame 13 {
                          n235 = control-ref of="藻密度"() -> (w435:refnum<vi>)
                          n236 = property class="Bool (严格)"(reference=w435) -> ("Label.Text"=w434:string)  [unwired: 1 in, 2 out]
                        }
                        frame 14 {
                          n237 = control-ref of="水位"() -> (w437:refnum<vi>)
                          n238 = property class="Bool (严格)"(reference=w437) -> ("Label.Text"=w436:string)  [unwired: 1 in, 2 out]
                        }
                        frame 15 {
                          n239 = control-ref of="流速"() -> (w439:refnum<vi>)
                          n240 = property class="Bool (严格)"(reference=w439) -> ("Label.Text"=w438:string)  [unwired: 1 in, 2 out]
                        }
                        frame 16 {
                          n241 = control-ref of="瞬时流量"() -> (w441:refnum<vi>)
                          n242 = property class="Bool (严格)"(reference=w441) -> ("Label.Text"=w440:string)  [unwired: 1 in, 2 out]
                        }
                        frame 17 {
                          n243 = control-ref of="累积流量"() -> (w443:refnum<vi>)
                          n244 = property class="Bool (严格)"(reference=w443) -> ("Label.Text"=w442:string)  [unwired: 1 in, 2 out]
                        }
                      }
                      n245 = global read "断电保存全局.vi" "数据发送协议"() -> (w269:enum16{"2005-212协议", "2017-212协议"})
                      n246 = call "主动发送数据生成Condition(子VI).vi"("数据发送协议"=w269, "database"=w271, "Label.Text"=w270, "数值"=w272) -> ("CONDITION"=w289:string)  [unwired: 7 in]
                      n247 = call "SQL查询.vi"("condition"=w289, "table输入"=w270, "database"=w271) -> ("error out"=w273:errorcluster, "data"=w285:string[][])  [unwired: 7 in]
                      n248 = Empty Array?(array=w285) -> (empty?=w288:bool)
                      n249 = call "短日期时间转长日期格式.vi"("data"=w285) -> ("输出数组"=w286:string[][])  [unwired: 10 in]
                      n250 = Not(x=w288) -> (.not. x?=w282:bool)
                      n251 = Index Array(array=w286, index (row)=w287, index (col)=w287) -> (element=w279:string)
                      n252 = global write "全局 水样时间.vi" "选择发送的参数"(w270) -> ()
                      n253 = flat-sequence {
                        tunnel: [w297] -> w284
                        tunnel: [w296] -> w283
                        tunnel: w282 -> [w297]
                        tunnel: w285 -> [w296]
                        tunnel: w272 -> [w291]
                        tunnel: w270 -> [w293]
                        tunnel: [w293] -> w280
                        tunnel: w279 -> [w292]
                        tunnel: [w292] -> w277
                        tunnel: [w291] -> w274
                        tunnel: w284 -> [w317]
                        tunnel: w283 -> [w320]
                        tunnel: [w319] -> w281
                        tunnel: w280 -> [w319]
                        tunnel: [w318] -> w278
                        tunnel: w277 -> [w318]
                        tunnel: [w317] -> w276
                        tunnel: [w316] -> w275
                        tunnel: w274 -> [w316]
                        tunnel: w281 -> [w376]
                        tunnel: w278 -> [w375]
                        tunnel: w276 -> [w373]
                        tunnel: w275 -> [w374]
                        frame #0 {
                          n254 = case shown="3" w291 {
                            tunnel: w296 -> [w298 w299 w300 w301 w302 w303 w304 w305 w306 w307 w308 w309 w310 w311 w312 w313 w314 w315]
                            frame 0, Default {
                              n255 = global write "全局 所有参数.vi" "CODMn"(w298) -> ()
                            }
                            frame 1 {
                              n256 = global write "全局 所有参数.vi" "CODCr"(w299) -> ()
                            }
                            frame 2 {
                              n257 = global write "全局 所有参数.vi" "DO"(w300) -> ()
                            }
                            frame 3 {
                              n258 = global write "全局 所有参数.vi" "铜"(w301) -> ()
                            }
                            frame 4 {
                              n259 = global write "全局 所有参数.vi" "PH"(w302) -> ()
                            }
                            frame 5 {
                              n260 = global write "全局 所有参数.vi" "氨氮"(w303) -> ()
                            }
                            frame 6 {
                              n261 = global write "全局 所有参数.vi" "电导率"(w304) -> ()
                            }
                            frame 7 {
                              n262 = global write "全局 所有参数.vi" "水温"(w305) -> ()
                            }
                            frame 8 {
                              n263 = global write "全局 所有参数.vi" "盐度"(w306) -> ()
                            }
                            frame 9 {
                              n264 = global write "全局 所有参数.vi" "浊度"(w307) -> ()
                            }
                            frame 10 {
                              n265 = global write "全局 所有参数.vi" "总氮"(w308) -> ()
                            }
                            frame 11 {
                              n266 = global write "全局 所有参数.vi" "总磷"(w309) -> ()
                            }
                            frame 12 {
                              n267 = global write "全局 所有参数.vi" "叶绿素"(w310) -> ()
                            }
                            frame 13 {
                              n268 = global write "全局 所有参数.vi" "藻密度"(w311) -> ()
                            }
                            frame 14 {
                              n269 = global write "全局 所有参数.vi" "水位"(w312) -> ()
                            }
                            frame 15 {
                              n270 = global write "全局 所有参数.vi" "流速"(w313) -> ()
                            }
                            frame 16 {
                              n271 = global write "全局 所有参数.vi" "瞬时流量"(w314) -> ()
                            }
                            frame 17 {
                              n272 = global write "全局 所有参数.vi" "累积流量"(w315) -> ()
                            }
                          }
                          n273 = global write "全局 小时数据发送次数.vi" "小时数据发送次数"(0 ("小时数据发送次数")) -> ()
                          n274 = global write "全局 数据发送重叠.vi" "数据接收超时指示灯"(FALSE ("数据接收超时指示灯")) -> ()
                          n275 = global write "全局1.vi" "枚举"(enum16{"返回请求应答", "上传数据", "返回执行结果"}."上传数据" ("枚举")) -> ()
                        }
                        frame #1 {
                          n276 = case shown="真" w317 {
                            tunnel: w320 -> [_ w323]
                            tunnel: w316 -> [_ w322]
                            tunnel: w316 -> [_ w321]
                            frame False {
                            }
                            frame True {
                              n277 = for {
                                tunnel: w323 -> [_] mode=indexing
                                tunnel: w322 -> [w341]
                                tunnel: w321 -> [w340]
                                # "实时数据的大小"
                                n278 = Wait (ms)(milliseconds to wait=u32 500 ("等待时间（毫秒）")) -> ()  [unwired: 1 out]
                                n279 = global write "全局 实时数据参数.vi" "实时数据参数"("水样测试" ("实时数据参数")) -> ()
                                n280 = Get Date/Time In Seconds() -> (seconds since 1Jan1904=w334:timestamp)
                                n281 = Format Date/Time String(time format string (%c)="%Y%m%d%H%M%S%3u" ("时间格式字符串(%c)"), seconds (now)=w334) -> (date/time string=w335:string)  [unwired: 1 in]
                                n282 = Search and Replace String(input string=w335, search string="." ("搜索字符串")) -> (result string=w337:string)  [unwired: 6 in, 3 out]
                                n283 = global read "断电保存全局.vi" "MN"() -> (w327:string)
                                n284 = global read "断电保存全局.vi" "PW"() -> (w326:string)
                                n285 = call "数据编码.vi"("table输入"="小时数据" ("新元素/子数组"), "QN"=w337, "MN"=w327, "PW"=w326) -> ("错误常量"=w324:errorcluster, "通讯包字符串"=w339:string)  [unwired: 10 in]
                                n286 = Build Array(w339) -> (w331:string[])
                                n287 = local write "发送报文显示"(w339) -> ()
                                n288 = call "发送数据记录到文档(子VI).vi"("数组"=w331) -> ()  [unwired: 9 in, 1 out]
                                n289 = call "通信状态入队列.vi"("错误输入（无错误）"=w324, "枚举"=enum16{"打开连接", "发送数据", "读取数据", "数据处理", "关闭连接"}."发送数据") -> ()  [unwired: 9 in, 1 out]
                                n290 = local read "判断数据反馈"() -> (w329:bool)
                                n291 = case shown="真" w329 {
                                tunnel: [_ w363] -> w338
                                tunnel: w339 -> [_ w362]
                                tunnel: w341 -> [_ w361]
                                frame False {
                                }
                                frame True {
                                n292 = case shown="0, 默认" w361 {
                                tunnel: [w365 _] -> w363
                                tunnel: w362 -> [w364 _]
                                frame 0, Default {
                                n293 = Empty String/Path?(string/path=w364) -> (empty?=w366:bool)
                                n294 = case shown="假" w366 {
                                tunnel: [w369 _] -> w365
                                tunnel: w364 -> [w368 _]
                                frame False {
                                n295 = local read "数据发送通道"() -> (w367:enum16{"TCP", "VISA"})
                                n296 = call "数据补发判定有限循环.vi"("数据输入"=w368, "数据发送通道"=w367) -> ("error out"=w369:errorcluster)  [unwired: 9 in]
                                }
                                frame True {
                                }
                                }
                                }
                                frame 14..17 {
                                }
                                }
                                }
                                }
                                n297 = local read "2011发送"() -> (w328:bool)
                                n298 = case shown="真" w328 {
                                tunnel: w340 -> [_ w354]
                                tunnel: w338 -> [_ w353]
                                frame False {
                                }
                                frame True {
                                n299 = global read "断电保存全局.vi" "MN"() -> (w345:string)
                                n300 = global read "断电保存全局.vi" "PW"() -> (w344:string)
                                n301 = global write "全局 实时数据参数.vi" "实时数据参数"("水样测试" ("实时数据参数")) -> ()
                                n302 = call "数据编码.vi"("table输入"="实时数据" ("新元素/子数组"), "错误常量 2"=w353, "MN"=w345, "PW"=w344) -> ("错误常量"=w346:errorcluster, "通讯包字符串"=w352:string)  [unwired: 10 in]
                                n303 = Build Array(w352) -> (w351:string[])
                                n304 = local write "发送报文显示"(w352) -> ()
                                n305 = call "发送数据记录到文档(子VI).vi"("数组"=w351) -> ()  [unwired: 9 in, 1 out]
                                n306 = call "通信状态入队列.vi"("错误输入（无错误）"=w346, "枚举"=enum16{"打开连接", "发送数据", "读取数据", "数据处理", "关闭连接"}."发送数据") -> ("错误输出"=w343:errorcluster)  [unwired: 9 in]
                                n307 = local read "判断数据反馈"() -> (w348:bool)
                                n308 = case shown="真" w348 {
                                tunnel: w352 -> [_ w357]
                                tunnel: w343 -> [_ w356]
                                tunnel: w354 -> [_ w355]
                                frame False {
                                }
                                frame True {
                                n309 = case shown="0, 默认" w355 {
                                tunnel: w357 -> [w360 _]
                                tunnel: w356 -> [w359 _]
                                frame 0, Default {
                                n310 = local read "数据发送通道"() -> (w358:enum16{"TCP", "VISA"})
                                n311 = call "数据补发判定有限循环.vi"("错误输入（无错误）"=w359, "数据输入"=w360, "数据发送通道"=w358) -> ()  [unwired: 8 in, 1 out]
                                }
                                frame 14..17 {
                                }
                                }
                                }
                                }
                                }
                                }
                              }
                            }
                          }
                        }
                        frame #2 {
                          n312 = global read "全局 数据发送重叠.vi" "数据接收超时指示灯"() -> (w370:bool)
                          n313 = Not(x=w370) -> (.not. x?=w371:bool)
                          n314 = Compound Arithmetic op=AND ("复合运算")(w371, w373) -> (w372:bool)
                          n315 = case shown="真" w372 {
                            tunnel: w375 -> [_ w379]
                            tunnel: w374 -> [_ w389]
                            tunnel: w376 -> [_ w380]
                            frame False {
                            }
                            frame True {
                              n316 = call "日期时间字符串转换分钟数加一.vi"("data[0]"=w379) -> ("日期/时间字符串"=w377:string)  [unwired: 10 in]
                              n317 = call "时间日期字符串至时间标识转换.vi"("时间日期字符串"=w377) -> ("时间标识"=w378:timestamp)  [unwired: 10 in]
                              n318 = call <vilib>:"Application Directory.vi"() -> ("Application Directory"=w381:path)
                              n319 = case shown="3" w389 {
                                tunnel: w377 -> [w390 w391 w392 w393 w394 w395 w396 w397 w398 w399 w400 w401 w402 w403 w404 w405 w406 w407]
                                frame 0, Default {
                                n320 = global write "全局 水样时间.vi" "time1"(w390) -> ()
                                }
                                frame 1 {
                                n321 = global write "全局 水样时间.vi" "time2"(w391) -> ()
                                }
                                frame 2 {
                                n322 = global write "全局 水样时间.vi" "time3"(w392) -> ()
                                }
                                frame 3 {
                                n323 = global write "全局 水样时间.vi" "time4"(w393) -> ()
                                }
                                frame 4 {
                                n324 = global write "全局 水样时间.vi" "time5"(w394) -> ()
                                }
                                frame 5 {
                                n325 = global write "全局 水样时间.vi" "time6"(w395) -> ()
                                }
                                frame 6 {
                                n326 = global write "全局 水样时间.vi" "time7"(w396) -> ()
                                }
                                frame 7 {
                                n327 = global write "全局 水样时间.vi" "time8"(w397) -> ()
                                }
                                frame 8 {
                                n328 = global write "全局 水样时间.vi" "time9"(w398) -> ()
                                }
                                frame 9 {
                                n329 = global write "全局 水样时间.vi" "time10"(w399) -> ()
                                }
                                frame 10 {
                                n330 = global write "全局 水样时间.vi" "time11"(w400) -> ()
                                }
                                frame 11 {
                                n331 = global write "全局 水样时间.vi" "time12"(w401) -> ()
                                }
                                frame 12 {
                                n332 = global write "全局 水样时间.vi" "time13"(w402) -> ()
                                }
                                frame 13 {
                                n333 = global write "全局 水样时间.vi" "time14"(w403) -> ()
                                }
                                frame 14 {
                                n334 = global write "全局 水样时间.vi" "time15"(w404) -> ()
                                }
                                frame 15 {
                                n335 = global write "全局 水样时间.vi" "time16"(w405) -> ()
                                }
                                frame 16 {
                                n336 = global write "全局 水样时间.vi" "time17"(w406) -> ()
                                }
                                frame 17 {
                                n337 = global write "全局 水样时间.vi" "time18"(w407) -> ()
                                }
                              }
                              n338 = Build Path(base path=w381, name or relative path="data\\Set.ini" ("名称或相对路径")) -> (appended path=w383:path)
                              n339 = call <vilib>:"Open Config Data.vi"("configuration file path"=w383) -> ("error out"=w385:errorcluster, "refnum"=w384:T8)  [unwired: 8 in, 1 out]
                              n340 = local write "数据发送起始时间"(w378) -> ()
                              n341 = call-poly <vilib>:"Write Key.vi"("section"="线程一数据搜索起始时间", "error in (no error)"=w385, "value"=w377, "key"=w380, "refnum"=w384) -> ("error out"=w387:errorcluster, "refnum out"=w386:T8)  [unwired: 4 in, 1 out]
                              n342 = call <vilib>:"Close Config Data.vi"("error in (no error)"=w387, "refnum"=w386) -> ()  [unwired: 8 in, 2 out]
                            }
                          }
                        }
                      }
                    }
                  }
                }
                "实时小时数据上传" <- w163
              }
              frame #1 {
                w444 = FALSE ("小时数据上传")
                n343 = local write "实时小时数据上传"(w444) -> ()
                n344 = global write "全局 数据发送重叠.vi" "主动上报数据中"(w444) -> ()
              }
            }
          }
          frame True {
            # "数据整点触发，整条发送"
          }
        }
      }
    }
  }
  n345 = while {
    stop <- FALSE stop-if-true
    # "数据整点触发，整条发送；数据自动重发设置"
    n346 = global read "断电保存全局.vi" "数据组合发送"() -> (w447:bool)
    n347 = case shown="真" "每周自动重发" {
      frame False {
      }
      frame True {
        (unwired) T1."00点"
        (unwired) T2."关闭"
        # "自动重发水样数据"
        n348 = Get Date/Time In Seconds() -> (seconds since 1Jan1904=w462:timestamp)
        n349 = Seconds To Date/Time(time stamp (now)=w462) -> (date time rec=w456:T9)  [unwired: 1 in]
        n350 = Unbundle By Name(w456) -> ("天数（周）"=w461:i32, "时"=w451:i32, "分"=w460:i32)
        n351 = Equal To 0?(x=w460) -> (x = 0?=w457:bool)
        n352 = Equal?(x=w461, y="重发日期") -> (x = y?=w459:bool)
        n353 = Equal?(x=w451, y="重发时间") -> (x = y?=w458:bool)
        n354 = Compound Arithmetic op=AND ("复合运算")(w459, w458, w457) -> (w455:bool)
        n355 = call <vilib>:"Boolean Crossing PtByPt.vi"("direction"=enum16{"either", "false-true", "true-false"}."false-true", "input"=w455) -> ("crossing"=w454:bool)  [unwired: 1 in]
        n356 = case shown="真" w454 {
          tunnel: w456 -> [_ w465]
          frame False {
          }
          frame True {
            n357 = local read "参数数值"() -> (w463:T5)
            n358 = Unbundle By Name(w465) -> ("日"=w468:i32)
            n359 = Cluster To Array(cluster=w463) -> (array=w470:bool[])
            n360 = Subtract(x=w468, y=7) -> (x-y=w466:i32)
            n361 = Bundle By Name(cluster=w465, "日"=w466) -> (w469:T9)
            n362 = Date/Time To Seconds(2:w469) -> (0:w464:timestamp)  [unwired: 1 in]
            n363 = for {
              tunnel: w470 -> [_] mode=indexing
              tunnel: w464 -> [w471]
              i -> [w472]
              n364 = Format Date/Time String(time format string (%c)="%Y/%m/%d %H:%M:%S" ("时间格式字符串(%c)"), seconds (now)=w471) -> (date/time string=w473:string)  [unwired: 1 in]
              n365 = case shown="16" w472 {
                tunnel: w473 -> [w475 w476 w477 w478 w479 w480 w481 w482 w483 w484 w485 w486 w487 w488 w489 w490 w491 w492]
                frame 0, Default {
                  n366 = global write "全局 水样时间.vi" "time1"(w475) -> ()
                }
                frame 1 {
                  n367 = global write "全局 水样时间.vi" "time2"(w476) -> ()
                }
                frame 2 {
                  n368 = global write "全局 水样时间.vi" "time3"(w477) -> ()
                }
                frame 3 {
                  n369 = global write "全局 水样时间.vi" "time4"(w478) -> ()
                }
                frame 4 {
                  n370 = global write "全局 水样时间.vi" "time5"(w479) -> ()
                }
                frame 5 {
                  n371 = global write "全局 水样时间.vi" "time6"(w480) -> ()
                }
                frame 6 {
                  n372 = global write "全局 水样时间.vi" "time7"(w481) -> ()
                }
                frame 7 {
                  n373 = global write "全局 水样时间.vi" "time8"(w482) -> ()
                }
                frame 8 {
                  n374 = global write "全局 水样时间.vi" "time9"(w483) -> ()
                }
                frame 9 {
                  n375 = global write "全局 水样时间.vi" "time10"(w484) -> ()
                }
                frame 10 {
                  n376 = global write "全局 水样时间.vi" "time11"(w485) -> ()
                }
                frame 11 {
                  n377 = global write "全局 水样时间.vi" "time12"(w486) -> ()
                }
                frame 12 {
                  n378 = global write "全局 水样时间.vi" "time13"(w487) -> ()
                }
                frame 13 {
                  n379 = global write "全局 水样时间.vi" "time14"(w488) -> ()
                }
                frame 14 {
                  n380 = global write "全局 水样时间.vi" "time15"(w489) -> ()
                }
                frame 15 {
                  n381 = global write "全局 水样时间.vi" "time16"(w490) -> ()
                }
                frame 16 {
                  n382 = global write "全局 水样时间.vi" "time17"(w491) -> ()
                }
                frame 17 {
                  n383 = global write "全局 水样时间.vi" "time18"(w492) -> ()
                }
              }
            }
          }
        }
      }
    }
    n384 = case shown="真" w447 {
      frame False {
      }
      frame True {
        n385 = Get Date/Time In Seconds() -> (seconds since 1Jan1904=w500:timestamp)
        n386 = Seconds To Date/Time(time stamp (now)=w500) -> (date time rec=w501:T9)  [unwired: 1 in]
        n387 = global read "断电保存全局.vi" "数据重发"() -> (w493:bool)
        n388 = Unbundle By Name(w501) -> ("分"=w499:i32)
        n389 = Equal?(x=w499, y=0) -> (x = y?=w497:bool)
        n390 = call <vilib>:"Boolean Crossing PtByPt.vi"("direction"=enum16{"either", "false-true", "true-false"}."false-true", "input"=w497) -> ("crossing"=w495:bool)  [unwired: 1 in]
        n391 = Or(x=w493, y=w495) -> (x .or. y?=w494:bool)
        n392 = case shown="真" w494 {
          frame False {
            n393 = global write "全局 数据发送重叠.vi" "主动上报数据中"(FALSE ("主动上报数据中")) -> ()
          }
          frame True {
            n394 = local read "数据发送通道"() -> (w505:enum16{"TCP", "VISA"})
            n395 = local read "MN"() -> (w504:string)
            n396 = local read "PW"() -> (w503:string)
            n397 = call "数据全参数一起发送整点触发.vi"("数据发送通道"=w505, "PW"=w503, "MN"=w504) -> ()  [unwired: 8 in]
          }
        }
      }
    }
    n398 = Wait (ms)(milliseconds to wait=u32 1000 ("等待时间（毫秒）")) -> ()  [unwired: 1 out]
  }
  n399 = Obtain Queue(name (unnamed)="STEP" ("名称（未命名）"), element data type=T6."初始化" ("枚举")) -> (queue out=w52:refnum<queue>)  [unwired: 3 in, 2 out]
  n400 = Insert Into Array(array=string[] [] ("tables"), index=0 ("索引"), new element="实时数据" ("新元素/子数组")) -> (w55:string[])
  n401 = Enqueue Element(queue=w52, element=T6."初始化" ("元素")) -> (queue out=w57:refnum<queue>)  [unwired: 2 in, 2 out]
  "主队列输出" <- w57
  n402 = Array Size(array=w55) -> (size(s)=w53:i32)
  n403 = while {
    stop <- FALSE stop-if-true
    # "心跳包"
    n404 = local read "数据发送通道"() -> (w513:enum16{"TCP", "VISA"})
    n405 = global read "全局 数据发送重叠.vi" "掉线指示灯"() -> (→"掉线指示":bool)
    n406 = Get Date/Time In Seconds() -> (seconds since 1Jan1904=w553:timestamp)
    n407 = local read "数据发送通道"() -> (w528:enum16{"TCP", "VISA"})
    n408 = local read "空闲时间"() -> (w545:dbl)
    n409 = case shown="\"VISA\"" w513 {
      tunnel: [w585 w588] -> w532
      tunnel: [w584 w586] -> w531
      frame "TCP", Default {
        n410 = local read "PORT"() -> (w584:string)
        n411 = local read "IP"() -> (w585:string)
      }
      frame "VISA" {
        n412 = local read "baud rate"() -> (w587:u32)
        n413 = local read "VISA resource name"() -> (w588:refnum<visa-resource-name>)
        n414 = Number To Decimal String(number=w587) -> (decimal integer string=w586:string)  [unwired: 1 in]
      }
    }
    n415 = Wait (ms)(milliseconds to wait=u32 1000 ("等待时间（毫秒）")) -> ()  [unwired: 1 out]
    n416 = global read "全局 数据发送重叠.vi" "主动上报数据中"() -> (w514:bool)
    n417 = local read "核查数据上传"() -> (w540:bool)
    n418 = local read "空闲时间"() -> (w576:dbl)
    n419 = local read "查询数据发送"() -> (w543:bool)
    n420 = Number To Decimal String(number=w545) -> (decimal integer string=→"空闲时间/s":string)  [unwired: 1 in]
    n421 = local read "站点设备"() -> (w533:string)
    n422 = local read "站点名称"() -> (w534:string)
    n423 = global read "全局 数据发送重叠.vi" "数据接收超时指示灯"() -> (→"数据接收超时指示灯":bool)
    n424 = local read "MN"() -> (w530:string)
    n425 = Format Date/Time String(time format string (%c)="%Y/%m/%d %H:%M:%S" ("时间格式字符串(%c)"), seconds (now)=w553) -> (date/time string=→"系统时间":string)  [unwired: 1 in]
    n426 = local read "PW"() -> (w529:string)
    n427 = local read "步骤"() -> (w570:T6)
    n428 = case shown="\"TCP\", 默认" w528 {
      frame "TCP", Default {
        w589 = TRUE ("可见")
        w590 = FALSE ("可见")
        n429 = property on="VISA resource name" class="VISAName"("Visible"=w590) -> ()  [unwired: 2 in, 2 out]
        n430 = property on="baud rate" class="DigNum (严格)"("Visible"=w590) -> ()  [unwired: 2 in, 2 out]
        n431 = property on="IP" class="Str"("Visible"=w589) -> ()  [unwired: 2 in, 2 out]
        n432 = property on="PORT" class="Str"("Visible"=w589) -> ()  [unwired: 2 in, 2 out]
      }
      frame "VISA" {
        w591 = TRUE ("可见")
        w592 = FALSE ("可见")
        n433 = property on="baud rate" class="DigNum (严格)"("Visible"=w591) -> ()  [unwired: 2 in, 2 out]
        n434 = property on="VISA resource name" class="VISAName"("Visible"=w591) -> ()  [unwired: 2 in, 2 out]
        n435 = property on="IP" class="Str"("Visible"=w592) -> ()  [unwired: 2 in, 2 out]
        n436 = property on="PORT" class="Str"("Visible"=w592) -> ()  [unwired: 2 in, 2 out]
      }
    }
    n437 = local read "数据发送协议"() -> (w526:enum16{"2005-212协议", "2017-212协议"})
    n438 = Not(x=w540) -> (.not. x?=w541:bool)
    n439 = Greater?(x=w576, y=30.0) -> (0:w574:bool)
    n440 = Not(x=w514) -> (.not. x?=w542:bool)
    n441 = property on="数据发送通道" class="Enum (严格)"("Visible"="锁") -> ()  [unwired: 2 in, 2 out]
    n442 = Not(x=w543) -> (.not. x?=w564:bool)
    n443 = Equal?(x=w570, y=T6."读取数据" ("步骤")) -> (x = y?=w568:bool)
    n444 = Bundle By Name(cluster=T4 {"站点"="", "设备"="", "IP"="", "PORT"="", "MN"="", "PW"=""} ("配置信息"), "站点"=w534, "设备"=w533, "IP"=w532, "PORT"=w531, "MN"=w530, "PW"=w529) -> (→"配置信息":T4)
    n445 = Select(t=T10."Enabled" ("禁用"), s="更改起始时间", f=T10."Disabled and Grayed Out" ("禁用")) -> (s? t:f=w556:T10)
    n446 = case shown="真" w574 {
      tunnel: w574 -> [_ w602]
      tunnel: [FALSE w602] -> w571
      frame False {
      }
      frame True {
        n447 = local read "QN"() -> (w600:string)
        n448 = local write "空闲时间"(0.0 ("空闲时间")) -> ()
        n449 = local read "MN"() -> (w599:string)
        n450 = local read "PW"() -> (w598:string)
        n451 = global read "断电保存全局.vi" "数据发送通道"() -> (w594:enum16{"TCP", "VISA"})
        n452 = call "数据编码.vi"("table输入"="心跳包", "QN"=w600, "MN"=w599, "PW"=w598) -> ("通讯包字符串"=w596:string)  [unwired: 10 in, 1 out]
        n453 = local write "发送报文显示"(w596) -> ()
        n454 = call "VISATCP组合选择发送.vi"("数据发送通道"=w594, "命令"="write", "写入缓冲区"=w596) -> ("错误输出"=w595:errorcluster)  [unwired: 9 in, 3 out]
        n455 = call <vilib>:"Clear Errors.vi"("error in (no error)"=w595) -> ()  [unwired: 5 in, 2 out]
      }
    }
    "心跳包" <- w571
    n456 = Select(t=T10."Enabled" ("禁用"), s="锁", f=T10."Disabled and Grayed Out" ("禁用")) -> (s? t:f=w519:T10)
    n457 = property on="数据发送起始时间" class="AbsTime (严格)"("DisabledEnum"=w556) -> ()  [unwired: 2 in, 2 out]
    n458 = global read "全局 时间2.vi" "跨度核查索引起始时间"() -> (→"跨度核查索引起始时间":string)
    n459 = case shown="\"2005-212协议\"" w526 {
      tunnel: ["32" ("设备编码MN") w579] -> w562
      frame "2005-212协议" {
      }
      frame "2017-212协议", Default {
        n460 = local read "系统编码选择框"() -> (w580:string)
        n461 = case shown="\"地表水质量监测\", 默认" w580 {
          tunnel: ["52" ("设备编码MN") "32" ("设备编码MN") "21" ("设备编码MN")] -> w579
          frame "污水排放过程监测" {
          }
          frame "地表水体污染源" {
          }
          frame "地表水质量监测", Default {
          }
        }
      }
    }
    n462 = global read "全局 时间2.vi" "标样核查索引起始时间"() -> (→"标样核查索引起始时间":string)
    n463 = global read "全局 时间2.vi" "零点核查索引起始时间"() -> (→"零点核查索引起始时间":string)
    n464 = global read "全局 时间2.vi" "加标回收索引起始时间"() -> (→"加标回收索引起始时间":string)
    n465 = property on="设置超时时间/min" class="DigNum (严格)"("DisabledEnum"=w519) -> ()  [unwired: 2 in, 2 out]
    n466 = property on="IP" class="Str"("DisabledEnum"=w519) -> ()  [unwired: 2 in, 2 out]
    n467 = property on="每周自动重发" class="Bool (严格)"("DisabledEnum"=w519) -> ()  [unwired: 2 in, 2 out]
    n468 = property on="PORT" class="Str"("DisabledEnum"=w519) -> ()  [unwired: 2 in, 2 out]
    n469 = local read "数据发送协议"() -> (w525:enum16{"2005-212协议", "2017-212协议"})
    n470 = local read "TCP服务端掉线计数"() -> (w548:i32)
    n471 = local read "1st Error to Convert"() -> (w551:i32)
    n472 = local read "TCP掉线时间节点"() -> (w547:string)
    n473 = property on="确定更改起始时间" class="Bool"("DisabledEnum"=w556) -> ()  [unwired: 2 in, 2 out]
    n474 = property on="MN" class="Str"("DisabledEnum"=w519) -> ()  [unwired: 2 in, 2 out]
    n475 = property on="PW" class="Str"("DisabledEnum"=w519) -> ()  [unwired: 2 in, 2 out]
    n476 = local read "元素"() -> (w549:string)
    n477 = local read "步骤"() -> (w550:T6)
    n478 = Equal?(x=w525, y=enum16{"2005-212协议", "2017-212协议"}."2017-212协议" ("数据发送协议")) -> (x = y?=w523:bool)
    n479 = Compound Arithmetic op=AND ("复合运算")(w523, w568, w564, w542, w541) -> (w565:bool)
    n480 = case shown="真" w565 {
      frame False {
      }
      frame True {
        n481 = local read "空闲时间"() -> (w605:dbl)
        n482 = Increment(x=w605) -> (x+1=→"空闲时间":dbl)
      }
    }
    n483 = property on="数据发送通道" class="Enum (严格)"("DisabledEnum"=w519) -> ()  [unwired: 2 in, 2 out]
    n484 = Bundle By Name(cluster=T3 {"1st Error to Convert "=54, "步骤 "=enum."打开连接", "元素"="实时数据", "TCP服务端掉线计数"=4, "TCP掉线时间节点"="2019/05/08 15:24:17"} ("状态信息"), "1st Error to Convert"=w551, "步骤"=w550, "元素"=w549, "TCP服务端掉线计数"=w548, "TCP掉线时间节点"=w547) -> (→"状态信息":T3)
    n485 = global read "全局1.vi" "通讯包字符串"() -> (w515:string)
    n486 = property on="重发时间" class="Enum (严格)"("DisabledEnum"=w519) -> ()  [unwired: 2 in, 2 out]
    n487 = property on="重发日期" class="Enum (严格)"("DisabledEnum"=w519) -> ()  [unwired: 2 in, 2 out]
    n488 = property on="VISA resource name" class="VISAName"("DisabledEnum"=w519) -> ()  [unwired: 2 in, 2 out]
    n489 = property on="判断数据反馈" class="Bool (严格)"("DisabledEnum"=w519) -> ()  [unwired: 2 in, 2 out]
    n490 = property on="baud rate" class="DigNum (严格)"("DisabledEnum"=w519) -> ()  [unwired: 2 in, 2 out]
    n491 = property on="数据发送协议" class="Enum (严格)"("DisabledEnum"=w519) -> ()  [unwired: 2 in, 2 out]
    n492 = property on="2011发送" class="Bool (严格)"("DisabledEnum"=w519) -> ()  [unwired: 2 in, 2 out]
    n493 = feedback #1(w515) -> (w516:string)
    n494 = feedback-in #1(w515) -> ()
    n495 = global write "全局1.vi" "系统编码ST"(w562) -> ()
    n496 = property on="日志、参数发送" class="Bool (严格)"("DisabledEnum"=w519) -> ()  [unwired: 2 in, 2 out]
    n497 = property on="数据组合发送" class="Bool (严格)"("DisabledEnum"=w519) -> ()  [unwired: 2 in, 2 out]
    n498 = Not Equal?(x=w515, y=w516) -> (x != y?=w517:bool)
    n499 = case shown="真" w517 {
      tunnel: w515 -> [_ w577]
      frame False {
      }
      frame True {
        n500 = local write "发送报文显示"(w577) -> ()
      }
    }
    n501 = global read "断电保存全局.vi" "日志、参数发送"() -> (w520:bool)
    n502 = global read "断电保存全局.vi" "数据组合发送"() -> (w518:bool)
    n503 = global read "全局1.vi" "读取报文显示"() -> (w509:string)
    n504 = global read "全局1.vi" "发送报文显示"() -> (w508:string)
    n505 = global read "断电保存全局.vi" "数据发送协议"() -> (w512:enum16{"2005-212协议", "2017-212协议"})
    n506 = global read "断电保存全局.vi" "判断数据反馈"() -> (w522:bool)
    n507 = global read "断电保存全局.vi" "数据发送通道"() -> (w511:enum16{"TCP", "VISA"})
    n508 = global read "断电保存全局.vi" "2011发送"() -> (w521:bool)
    n509 = local read "QN"() -> (w510:string)
    n510 = local write "日志、参数发送"(w520) -> ()
    n511 = local write "数据组合发送"(w518) -> ()
    n512 = local write "读取报文显示"(w509) -> ()
    n513 = local write "数据发送协议"(w512) -> ()
    n514 = local write "判断数据反馈"(w522) -> ()
    n515 = local write "数据发送通道"(w511) -> ()
    n516 = local write "发送报文显示"(w508) -> ()
    n517 = local write "2011发送"(w521) -> ()
    n518 = global write "全局1.vi" "QN"(w510) -> ()
    n519 = global write "断电保存全局.vi" "MN"("MN") -> ()
    n520 = global write "断电保存全局.vi" "PW"("PW") -> ()
  }
  n521 = while {
    stop <- FALSE stop-if-true
    # "定期释放缓存"
    n522 = Wait (ms)(milliseconds to wait=u32 600000 ("等待时间（毫秒）")) -> ()  [unwired: 1 out]
    n523 = dll-call lib="PTH2aabs F\tgitkrakenCC6平台数采程序 - V2.0.1（正式修改迭代版）dataFreeMem.dll" fn="FreeMem"() -> ()  [unwired: 4 in, 2 out]
  }
  n524 = while {
    stop <- FALSE stop-if-true
    n525 = event shown="[15] \"返回主界面\": 值改变" {
      selector: _ -> [_ _ _ _ _ _ _ _ _ _ _ _ _ _ _ _]
      dyn-events: _ -> [_ _ _ _ _ _ _ _ _ _ _ _ _ _ _ _]
      timeout: _ -> [_ _ _ _ _ _ _ _ _ _ _ _ _ _ _ _]
      event Timeout {
        n526 = event-data() -> ()  [unwired: 1 in, 2 out]
      }
      event "站点名称", "站点设备", "IP", "PORT", "MN", "PW", "VISA resource name", "baud rate": Value Change {
        w611 = "线程一自主部署站点保存"
        # "TCP服务器端口掉线"
        n527 = event-data() -> ()  [unwired: 1 in, 6 out]
        n528 = call <vilib>:"Application Directory.vi"() -> ("Application Directory"=w653:path)
        n529 = local read "站点名称"() -> (w632:string)
        n530 = Build Path(base path=w653, name or relative path="data\\Set.ini" ("名称或相对路径")) -> (appended path=w651:path)
        n531 = call <vilib>:"Open Config Data.vi"("configuration file path"=w651) -> ("error out"=w649:errorcluster, "refnum"=w650:T8)  [unwired: 8 in, 1 out]
        n532 = local read "站点设备"() -> (w631:string)
        n533 = call-poly <vilib>:"Write Key.vi"("section"=w611, "error in (no error)"=w649, "value"=w632, "key"="站点名称", "refnum"=w650) -> ("error out"=w646:errorcluster, "refnum out"=w647:T8)  [unwired: 4 in, 1 out]
        n534 = call-poly <vilib>:"Write Key.vi"("section"=w611, "error in (no error)"=w646, "value"=w631, "key"="站点设备", "refnum"=w647) -> ("error out"=w643:errorcluster, "refnum out"=w644:T8)  [unwired: 4 in, 1 out]
        n535 = local read "IP"() -> (w630:string)
        n536 = call-poly <vilib>:"Write Key.vi"("section"=w611, "error in (no error)"=w643, "value"=w630, "key"="IP", "refnum"=w644) -> ("error out"=w641:errorcluster, "refnum out"=w642:T8)  [unwired: 4 in, 1 out]
        n537 = local read "PORT"() -> (w629:string)
        n538 = call-poly <vilib>:"Write Key.vi"("section"=w611, "error in (no error)"=w641, "value"=w629, "key"="PORT", "refnum"=w642) -> ("error out"=w639:errorcluster, "refnum out"=w640:T8)  [unwired: 4 in, 1 out]
        n539 = local read "MN"() -> (w623:string)
        n540 = call-poly <vilib>:"Write Key.vi"("section"=w611, "error in (no error)"=w639, "value"=w623, "key"="MN", "refnum"=w640) -> ("error out"=w624:errorcluster, "refnum out"=w627:T8)  [unwired: 4 in, 1 out]
        n541 = local read "PW"() -> (w625:string)
        n542 = call-poly <vilib>:"Write Key.vi"("section"=w611, "error in (no error)"=w624, "value"=w625, "key"="PW", "refnum"=w627) -> ("error out"=w612:errorcluster, "refnum out"=w613:T8)  [unwired: 4 in, 1 out]
        n543 = local read "VISA resource name"() -> (w619:refnum<visa-resource-name>)
        n544 = local read "主队列输出"() -> (w638:refnum<queue>)
        n545 = call-poly <vilib>:"Write Key.vi"("section"=w611, "error in (no error)"=w612, "value"=w619, "key"="VISA", "refnum"=w613) -> ("error out"=w618:errorcluster, "refnum out"=w615:T8)  [unwired: 4 in, 1 out]
        n546 = local read "baud rate"() -> (w617:u32)
        n547 = Flush Queue(queue=w638) -> (queue out=w637:refnum<queue>)  [unwired: 1 in, 2 out]
        n548 = call-poly <vilib>:"Write Key.vi"("section"=w611, "error in (no error)"=w618, "value"=w617, "key"="BAUDRATE", "refnum"=w615) -> ("error out"=w609:errorcluster, "refnum out"=w610:T8)  [unwired: 4 in, 1 out]
        n549 = local read "数据发送通道"() -> (w622:enum16{"TCP", "VISA"})
        n550 = call <vilib>:"Close Config Data.vi"("error in (no error)"=w609, "refnum"=w610) -> ()  [unwired: 8 in, 2 out]
        n551 = call "VISATCP组合选择发送.vi"("数据发送通道"=w622, "命令"="close") -> ("错误输出"=w620:errorcluster)  [unwired: 10 in, 3 out]
        n552 = Enqueue Element(queue=w637, element=T6."初始化" ("元素"), timeout in ms (-1)=1000 ("超时毫秒(-1)")) -> ()  [unwired: 1 in, 3 out]
        n553 = call <vilib>:"Clear Errors.vi"("error in (no error)"=w620) -> ()  [unwired: 5 in, 2 out]
      }
      event "确定": Value Change {
        w658 = "线程一自主部署站点保存"
        # "TCP服务器端口掉线"
        n554 = event-data() -> ()  [unwired: 1 in, 6 out]
        n555 = call <vilib>:"Application Directory.vi"() -> ("Application Directory"=w691:path)
        n556 = local read "站点名称"() -> (w686:string)
        n557 = Build Path(base path=w691, name or relative path="data\\Set.ini" ("名称或相对路径")) -> (appended path=w689:path)
        n558 = call <vilib>:"Open Config Data.vi"("configuration file path"=w689) -> ("error out"=w687:errorcluster, "refnum"=w688:T8)  [unwired: 8 in, 1 out]
        n559 = local read "站点设备"() -> (w681:string)
        n560 = call-poly <vilib>:"Write Key.vi"("section"=w658, "error in (no error)"=w687, "value"=w686, "key"="站点名称", "refnum"=w688) -> ("error out"=w683:errorcluster, "refnum out"=w684:T8)  [unwired: 4 in, 1 out]
        n561 = call-poly <vilib>:"Write Key.vi"("section"=w658, "error in (no error)"=w683, "value"=w681, "key"="站点设备", "refnum"=w684) -> ("error out"=w679:errorcluster, "refnum out"=w680:T8)  [unwired: 4 in, 1 out]
        n562 = local read "IP"() -> (w674:string)
        n563 = local read "PORT"() -> (w673:string)
        n564 = call-poly <vilib>:"Write Key.vi"("section"=w658, "error in (no error)"=w679, "value"=w674, "key"="IP", "refnum"=w680) -> ("error out"=w677:errorcluster, "refnum out"=w678:T8)  [unwired: 4 in, 1 out]
        n565 = call-poly <vilib>:"Write Key.vi"("section"=w658, "error in (no error)"=w677, "value"=w673, "key"="PORT", "refnum"=w678) -> ("error out"=w669:errorcluster, "refnum out"=w670:T8)  [unwired: 4 in, 1 out]
        n566 = local read "MN"() -> (w666:string)
        n567 = call-poly <vilib>:"Write Key.vi"("section"=w658, "error in (no error)"=w669, "value"=w666, "key"="MN", "refnum"=w670) -> ("error out"=w667:errorcluster, "refnum out"=w668:T8)  [unwired: 4 in, 1 out]
        n568 = local read "PW"() -> (w665:string)
        n569 = call-poly <vilib>:"Write Key.vi"("section"=w658, "error in (no error)"=w667, "value"=w665, "key"="PW", "refnum"=w668) -> ("error out"=w663:errorcluster, "refnum out"=w664:T8)  [unwired: 4 in, 1 out]
        n570 = call <vilib>:"Close Config Data.vi"("error in (no error)"=w663, "refnum"=w664) -> ("error out"=w657:errorcluster)  [unwired: 8 in, 1 out]
        n571 = local read "主队列输出"() -> (w662:refnum<queue>)
        n572 = local read "数据发送通道"() -> (w656:enum16{"TCP", "VISA"})
        n573 = call "VISATCP组合选择发送.vi"("数据发送通道"=w656, "命令"="close") -> ("错误输出"=w654:errorcluster)  [unwired: 10 in, 3 out]
        n574 = Flush Queue(queue=w662) -> (queue out=w661:refnum<queue>)  [unwired: 1 in, 2 out]
        n575 = case shown="错误" w657 {
          frame No Error {
            n576 = One Button Dialog(message="保存成功" ("消息"), button name ("OK")="确定" ("按钮名称（“确定”）")) -> ()  [unwired: 1 out]
          }
          frame Error {
            n577 = One Button Dialog(message="保存失败" ("消息"), button name ("OK")="确定" ("按钮名称（“确定”）")) -> ()  [unwired: 1 out]
          }
        }
        n578 = call <vilib>:"Clear Errors.vi"("error in (no error)"=w654) -> ()  [unwired: 5 in, 2 out]
        n579 = Enqueue Element(queue=w661, element=T6."初始化" ("元素"), timeout in ms (-1)=1000 ("超时毫秒(-1)")) -> ()  [unwired: 1 in, 3 out]
      }
      event "参数配置": Value Change {
        n580 = event-data() -> ()  [unwired: 1 in, 6 out]
        n581 = property on="窗格" class="Pane"("Origin"=T11 {"Horizontal"=0, "Vertical"=1000} ("原点")) -> ()  [unwired: 2 in, 2 out]
      }
      event "返回": Value Change {
        n582 = event-data() -> ()  [unwired: 1 in, 6 out]
        n583 = property on="窗格" class="Pane"("Origin"=T11 {"Horizontal"=0, "Vertical"=0} ("原点")) -> ()  [unwired: 2 in, 2 out]
      }
      event "系统编码选择框": Value Change {
        n584 = event-data() -> ()  [unwired: 1 in, 6 out]
        n585 = call <vilib>:"Application Directory.vi"() -> ("Application Directory"=w706:path)
        n586 = Build Path(base path=w706, name or relative path="data\\Set.ini" ("名称或相对路径")) -> (appended path=w707:path)
        n587 = call <vilib>:"Open Config Data.vi"("configuration file path"=w707) -> ("error out"=w703:errorcluster, "refnum"=w704:T8)  [unwired: 8 in, 1 out]
        n588 = call-poly <vilib>:"Write Key.vi"("section"="系统编码选择", "error in (no error)"=w703, "value"="系统编码选择框", "key"="系统编码", "refnum"=w704) -> ("error out"=w701:errorcluster, "refnum out"=w702:T8)  [unwired: 4 in, 1 out]
        n589 = call <vilib>:"Close Config Data.vi"("error in (no error)"=w701, "refnum"=w702) -> ()  [unwired: 8 in, 2 out]
      }
      event "判断数据反馈", "2011发送", "日志、参数发送", "数据组合发送", "数据发送通道", "数据发送协议": Value Change {
        n590 = event-data() -> ()  [unwired: 1 in, 6 out]
        n591 = flat-sequence {
          frame #0 {
            n592 = global write "断电保存全局.vi" "日志、参数发送"("日志、参数发送") -> ()
            n593 = global write "断电保存全局.vi" "判断数据反馈"("判断数据反馈") -> ()
            n594 = global write "断电保存全局.vi" "数据发送通道"("数据发送通道") -> ()
            n595 = global write "断电保存全局.vi" "2011发送"("2011发送") -> ()
            n596 = global write "断电保存全局.vi" "数据组合发送"("数据组合发送") -> ()
            n597 = global write "断电保存全局.vi" "数据发送协议"("数据发送协议") -> ()
          }
          frame #1 {
            n598 = call <vilib>:"Application Directory.vi"() -> ("Application Directory"=w714:path)
            n599 = Build Path(base path=w714, name or relative path="data\\sys.ini" ("名称或相对路径")) -> (appended path=w716:path)
            n600 = call <vilib>:"Open Config Data.vi"("configuration file path"=w716) -> ("error out"=w720:errorcluster, "refnum"=w717:T8)  [unwired: 8 in, 1 out]
            n601 = vi-ref "断电保存全局.vi"() -> (w718:refnum<vi>)
            n602 = call <userlib>:"Write Panel to INI__ogtk.vi"("error in (no error)"=w720, "VI ref"=w718, "refnum"=w717) -> ("error out"=w721:errorcluster, "refnum out"=w719:T8)  [unwired: 7 in]
            n603 = call <vilib>:"Close Config Data.vi"("error in (no error)"=w721, "refnum"=w719) -> ("error out"=w726:errorcluster, "file path"=w727:path)  [unwired: 8 in]
            n604 = Open/Create/Replace File(file path (use dialog)=w727, error in=w726) -> (refnum out=w723:refnum<file>, error out=w722:errorcluster)  [unwired: 4 in, 1 out]
            n605 = Flush File(refnum=w723, error in=w722) -> (refnum out=w724:refnum<file>, error out=w725:errorcluster)
            n606 = Close File(refnum=w724, error in=w725) -> ()  [unwired: 2 out]
          }
        }
      }
      event "每周自动重发": Value Change {
        n607 = event-data() -> ()  [unwired: 1 in, 6 out]
        n608 = call <vilib>:"Application Directory.vi"() -> ("Application Directory"=w736:path)
        n609 = Build Path(base path=w736, name or relative path="data\\Set.ini" ("名称或相对路径")) -> (appended path=w737:path)
        n610 = local read "每周自动重发"() -> (w728:bool)
        n611 = call <vilib>:"Open Config Data.vi"("configuration file path"=w737) -> ("error out"=w733:errorcluster, "refnum"=w734:T8)  [unwired: 8 in, 1 out]
        n612 = call-poly <vilib>:"Write Key.vi"("section"="线程一数据重发功能", "error in (no error)"=w733, "value"=w728, "key"="重发功能", "refnum"=w734) -> ("error out"=w731:errorcluster, "refnum out"=w732:T8)  [unwired: 4 in, 1 out]
        n613 = call <vilib>:"Close Config Data.vi"("error in (no error)"=w731, "refnum"=w732) -> ()  [unwired: 8 in, 2 out]
      }
      event "重发日期": Value Change {
        n614 = event-data() -> ()  [unwired: 1 in, 6 out]
        n615 = call <vilib>:"Application Directory.vi"() -> ("Application Directory"=w746:path)
        n616 = Build Path(base path=w746, name or relative path="data\\Set.ini" ("名称或相对路径")) -> (appended path=w747:path)
        n617 = local read "重发日期"() -> (w738:T2)
        n618 = call <vilib>:"Open Config Data.vi"("configuration file path"=w747) -> ("error out"=w743:errorcluster, "refnum"=w744:T8)  [unwired: 8 in, 1 out]
        n619 = call-poly <vilib>:"Write Key.vi"("section"="线程一数据重发功能", "error in (no error)"=w743, "value"=w738, "key"="重发日期", "refnum"=w744) -> ("error out"=w741:errorcluster, "refnum out"=w742:T8)  [unwired: 4 in, 1 out]
        n620 = call <vilib>:"Close Config Data.vi"("error in (no error)"=w741, "refnum"=w742) -> ()  [unwired: 8 in, 2 out]
      }
      event "重发时间": Value Change {
        n621 = event-data() -> ()  [unwired: 1 in, 6 out]
        n622 = call <vilib>:"Application Directory.vi"() -> ("Application Directory"=w756:path)
        n623 = Build Path(base path=w756, name or relative path="data\\Set.ini" ("名称或相对路径")) -> (appended path=w757:path)
        n624 = local read "重发时间"() -> (w748:T1)
        n625 = call <vilib>:"Open Config Data.vi"("configuration file path"=w757) -> ("error out"=w753:errorcluster, "refnum"=w754:T8)  [unwired: 8 in, 1 out]
        n626 = call-poly <vilib>:"Write Key.vi"("section"="线程一数据重发功能", "error in (no error)"=w753, "value"=w748, "key"="重发时间", "refnum"=w754) -> ("error out"=w751:errorcluster, "refnum out"=w752:T8)  [unwired: 4 in, 1 out]
        n627 = call <vilib>:"Close Config Data.vi"("error in (no error)"=w751, "refnum"=w752) -> ()  [unwired: 8 in, 2 out]
      }
      event "确定更改起始时间": Value Change {
        n628 = event-data() -> ()  [unwired: 1 in, 6 out]
        n629 = local write "更改起始时间"(FALSE ("更改起始时间")) -> ()
        n630 = Two Button Dialog(message="确定以当前设置时间作为数据索引起始时间？" ("消息")) -> (T button?=w759:bool)  [unwired: 2 in]
        n631 = case shown="真" w759 {
          frame False {
          }
          frame True {
            n632 = local read "参数数值"() -> (w764:T5)
            n633 = global write "断电保存全局.vi" "数据重发"(TRUE ("数据重发")) -> ()
            n634 = Cluster To Array(cluster=w764) -> (array=w765:bool[])
            n635 = for {
              tunnel: w765 -> [_] mode=indexing
              tunnel: [w775] -> w763
              i -> [w776]
              n636 = Format Date/Time String(time format string (%c)="%Y/%m/%d %H:%M:%S" ("时间格式字符串(%c)"), seconds (now)="数据发送起始时间") -> (date/time string=w775:string)  [unwired: 1 in]
              n637 = global write "断电保存全局.vi" "数据重发时间戳"(w775) -> ()
              n638 = case shown="0, 默认" w776 {
                tunnel: w775 -> [w779 w780 w781 w782 w783 w784 w785 w786 w787 w788 w789 w790 w791 w792 w793 w794 w795 w796]
                frame 0, Default {
                  n639 = global write "全局 水样时间.vi" "time1"(w779) -> ()
                }
                frame 1 {
                  n640 = global write "全局 水样时间.vi" "time2"(w780) -> ()
                }
                frame 2 {
                  n641 = global write "全局 水样时间.vi" "time3"(w781) -> ()
                }
                frame 3 {
                  n642 = global write "全局 水样时间.vi" "time4"(w782) -> ()
                }
                frame 4 {
                  n643 = global write "全局 水样时间.vi" "time5"(w783) -> ()
                }
                frame 5 {
                  n644 = global write "全局 水样时间.vi" "time6"(w784) -> ()
                }
                frame 6 {
                  n645 = global write "全局 水样时间.vi" "time7"(w785) -> ()
                }
                frame 7 {
                  n646 = global write "全局 水样时间.vi" "time8"(w786) -> ()
                }
                frame 8 {
                  n647 = global write "全局 水样时间.vi" "time9"(w787) -> ()
                }
                frame 9 {
                  n648 = global write "全局 水样时间.vi" "time10"(w788) -> ()
                }
                frame 10 {
                  n649 = global write "全局 水样时间.vi" "time11"(w789) -> ()
                }
                frame 11 {
                  n650 = global write "全局 水样时间.vi" "time12"(w790) -> ()
                }
                frame 12 {
                  n651 = global write "全局 水样时间.vi" "time13"(w791) -> ()
                }
                frame 13 {
                  n652 = global write "全局 水样时间.vi" "time14"(w792) -> ()
                }
                frame 14 {
                  n653 = global write "全局 水样时间.vi" "time15"(w793) -> ()
                }
                frame 15 {
                  n654 = global write "全局 水样时间.vi" "time16"(w794) -> ()
                }
                frame 16 {
                  n655 = global write "全局 水样时间.vi" "time17"(w795) -> ()
                }
                frame 17 {
                  n656 = global write "全局 水样时间.vi" "time18"(w796) -> ()
                }
              }
            }
            n657 = global read "断电保存全局.vi" "数据组合发送"() -> (w761:bool)
            n658 = case shown="假" w761 {
              tunnel: w763 -> [w766 _]
              frame False {
                n659 = global write "全局 时间2.vi" "跨度核查索引起始时间"(w766) -> ()
                n660 = global write "全局 时间2.vi" "标样核查索引起始时间"(w766) -> ()
                n661 = global write "全局 时间2.vi" "零点核查索引起始时间"(w766) -> ()
                n662 = global write "全局 时间2.vi" "加标回收索引起始时间"(w766) -> ()
                n663 = for {
                  N: 5 -> [_]
                  tunnel: w766 -> [w768]
                  i -> [w769]
                  n664 = case shown="1" w769 {
                    tunnel: w768 -> [w770 w771 w772 w773 w774]
                    frame 0, Default {
                      n665 = global write "全局 时间2.vi" "氨氮跨度核查索引起始时间"(w770) -> ()
                      n666 = global write "全局 时间2.vi" "氨氮零点核查索引起始时间"(w770) -> ()
                    }
                    frame 1 {
                      n667 = global write "全局 时间2.vi" "总氮跨度核查索引起始时间"(w771) -> ()
                      n668 = global write "全局 时间2.vi" "总氮零点核查索引起始时间"(w771) -> ()
                    }
                    frame 2 {
                      n669 = global write "全局 时间2.vi" "总磷跨度核查索引起始时间"(w772) -> ()
                      n670 = global write "全局 时间2.vi" "总磷零点核查索引起始时间"(w772) -> ()
                    }
                    frame 3 {
                      n671 = global write "全局 时间2.vi" "CODMn跨度核查索引起始时间"(w773) -> ()
                      n672 = global write "全局 时间2.vi" "CODMn零点核查索引起始时间"(w773) -> ()
                    }
                    frame 4 {
                      n673 = global write "全局 时间2.vi" "CODCr跨度核查索引起始时间"(w774) -> ()
                      n674 = global write "全局 时间2.vi" "CODCr零点核查索引起始时间"(w774) -> ()
                    }
                  }
                }
              }
              frame True {
              }
            }
          }
        }
      }
      event "开机启动": Value Change {
        n675 = event-data() -> ("NewVal"=w797:bool)  [unwired: 1 in, 5 out]
        n676 = case shown="假" w797 {
          frame False {
            n677 = Two Button Dialog(message="是否删除开机启动" ("消息"), 1:"否" ("F按钮名称（“取消”）"), 2:"是" ("T按钮名称（“确定”）")) -> (T button?=w798:bool)
            n678 = case shown="真" w798 {
              frame False {
              }
              frame True {
                n679 = call <vilib>:"Application Directory.vi"() -> ("Application Directory"=w803:path)
                n680 = call "删除启动项.vi"("启动文件路径"=w803) -> ("删除标记"=w802:bool)  [unwired: 9 in, 1 out]
                n681 = case shown="假" w802 {
                  tunnel: ["删除开机启动失败" ("T按钮名称（“确定”）") "删除开机启动成功" ("T按钮名称（“确定”）")] -> w804
                  frame False {
                  }
                  frame True {
                  }
                }
                n682 = One Button Dialog(message=w804) -> ()  [unwired: 1 in, 1 out]
              }
            }
          }
          frame True {
            n683 = Two Button Dialog(message="是否添加开机启动" ("消息"), 1:"否" ("F按钮名称（“取消”）"), 2:"是" ("T按钮名称（“确定”）")) -> (T button?=w807:bool)
            n684 = case shown="真" w807 {
              frame False {
              }
              frame True {
                n685 = call <vilib>:"Application Directory.vi"() -> ("Application Directory"=w813:path)
                n686 = call "添加启动项.vi"("启动文件路径"=w813) -> ("添加成功标记"=w812:bool)  [unwired: 9 in, 1 out]
                n687 = case shown="真" w812 {
                  tunnel: ["添加开机启动失败" ("T按钮名称（“确定”）") "添加开机启动成功" ("T按钮名称（“确定”）")] -> w811
                  frame False {
                  }
                  frame True {
                  }
                }
                n688 = One Button Dialog(message=w811) -> ()  [unwired: 1 in, 1 out]
              }
            }
          }
        }
      }
      event "IP": Mouse Down {
        n689 = event-data() -> ("CtlRef"=w816:refnum<vi>)  [unwired: 1 in, 5 out]
        n690 = property class="Str" props=["Value"](reference=w816) -> ()  [unwired: 1 in, 3 out]
        n691 = local read "IP"() -> (w818:string)
        n692 = call "IP键盘.vi"("OldNumber"=w818) -> ("NewNumber"=w817:string)
        n693 = local write "IP"(w817) -> ()
      }
      event "PORT": Mouse Down {
        n694 = event-data() -> ()  [unwired: 1 in, 6 out]
        n695 = local read "PORT"() -> (w820:string)
        n696 = call "IP键盘.vi"("OldNumber"=w820) -> ("NewNumber"=w819:string)
        n697 = local write "PORT"(w819) -> ()
      }
      event "查询质控数据起始时间": Value Change {
        n698 = event-data() -> ()  [unwired: 1 in, 6 out]
        n699 = property on="窗格" class="Pane"("Origin"=T11 {"Horizontal"=1000, "Vertical"=0} ("原点")) -> ()  [unwired: 2 in, 2 out]
      }
      event "返回主界面": Value Change {
        n700 = event-data() -> ()  [unwired: 1 in, 6 out]
        n701 = property on="窗格" class="Pane"("Origin"=T11 {"Horizontal"=0, "Vertical"=0} ("原点")) -> ()  [unwired: 2 in, 2 out]
      }
    }
  }
  n702 = while {
    shift-right: [w823] -> _
    shift-left: errorcluster {"status"=FALSE, "code"=0, "source"=""} ("error out") -> [w835]
    shift-right: [w832] -> _
    shift-left: _ -> [w831]
    tunnel: w57 -> [w834]
    tunnel: w55 -> [w830]
    shift-right: [w828] -> _
    shift-left: w37 -> [w829]
    tunnel: w53 -> [w827]
    shift-right: [w825] -> _
    shift-left: w37 -> [w826]
    stop <- FALSE stop-if-true
    n703 = case shown="无错误" w835 {
      selector: w835 -> [w853 w1021]
      tunnel: [w836 w1024] -> w823
      tunnel: w834 -> [w852 w1019]
      tunnel: [w837 w1023] -> w832
      tunnel: w831 -> [w849 w1023]
      tunnel: w830 -> [w848 _]
      tunnel: w829 -> [w843 w1022]
      tunnel: [w846 w1022] -> w828
      tunnel: w827 -> [w845 _]
      tunnel: w826 -> [w840 w1018]
      tunnel: [w839 w1018] -> w825
      frame No Error {
        n704 = Less?(x=w843, y=w845) -> (x < y?=w844:bool)
        n705 = Dequeue Element(queue=w852) -> (queue out=w850:refnum<queue>, element=w851:T6)  [unwired: 2 in, 2 out]
        "步骤" <- w851
        n706 = Select(t=w843, s=w844, f=0) -> (s? t:f=w842:i32)
        n707 = local read "元素"() -> (w838:string)
        n708 = Index Array(array=w848, index=w842) -> (element=→"元素":string)
        n709 = case shown="\"发送数据\"" w851 {
          tunnel: w853 -> [w860 _ w883 w890 w933 w1015]
          tunnel: w850 -> [w857 w874 w878 _ w931 w1013]
          tunnel: [w860 w862 w883 w888 w930 w1015] -> w836
          tunnel: [string[] [] ("待发送第一条数据") w876 _ w913 w934 _] -> w837
          tunnel: w849 -> [_ w876 _ w913 w934 w1014]
          tunnel: w838 -> [_ _ _ _ _ w1008]
          tunnel: w842 -> [w858 w873 w882 w914 w935 w1004]
          tunnel: [w858 w873 w881 w914 w935 w1005] -> w846
          tunnel: w840 -> [w855 w871 w880 _ w926 w1002]
          tunnel: [w855 w871 w880 0 ("索引") w929 w1002] -> w839
          frame "初始化", Default {
            n710 = Enqueue Element(queue=w857, element=T6."打开连接" ("元素"), timeout in ms (-1)=1000 ("超时毫秒(-1)")) -> ()  [unwired: 1 in, 3 out]
          }
          frame "打开连接" {
            (unwired) "47.98.43.76"
            # "和时通数据接入平台端接收IP端口号，61.191.22.195:10003。"
            # "47.98.43.76:6666"
            n711 = Enqueue Element(queue=w874, element=T6."表格比对" ("元素"), timeout in ms (-1)=1000 ("超时毫秒(-1)")) -> ()  [unwired: 1 in, 3 out]
            n712 = local read "数据发送通道"() -> (w861:enum16{"TCP", "VISA"})
            n713 = call "VISATCP组合选择发送.vi"("IP"="IP", "数据发送通道"=w861, "命令"="open", "PORT"="PORT", "VISA resource name"="VISA resource name", "baud rate"="baud rate") -> ("错误输出"=w862:errorcluster)  [unwired: 6 in, 3 out]
            n714 = Unbundle By Name(w862) -> ("status"=w870:bool, "code"=→"1st Error to Convert":i32)
            n715 = Not(x=w870) -> (.not. x?=→"通信状态":bool)
          }
          frame "表格比对" {
            n716 = Enqueue Element(queue=w878, element=T6."读取数据" ("元素"), timeout in ms (-1)=1000 ("超时毫秒(-1)")) -> ()  [unwired: 1 in, 3 out]
            n717 = Increment(x=w882) -> (x+1=w881:i32)
          }
          frame "读取数据" {
            # "设置测量时间间隔"
            # "1000设置超时时间和重发次数\n1011提取监测仪表时间\n1012设置监测仪表时间\n1014提取数采仪时间\n1015设置数采仪时间\n1061提取实时数据间隔\n1062设置实时数据间隔\n1072设置数采仪访问密码"
            # "6分钟掉线重连"
            n718 = local write "查询数据发送"(FALSE ("数据正在发送")) -> ()
            n719 = global write "全局 数据发送重叠.vi" "掉线指示灯"(FALSE ("数据发送重叠")) -> ()
            n720 = property on="TCP服务端掉线计数" class="DigNum (严格)"("Value"=0 ("TCP服务端掉线计数")) -> ()  [unwired: 2 in, 2 out]
            n721 = local read "数据发送通道"() -> (w892:enum16{"TCP", "VISA"})
            n722 = call "VISATCP组合选择发送.vi"("数据发送通道"=w892, "命令"="read", "error in (no error)"=w890) -> ("读取缓冲区"=w889:string, "错误输出"=w888:errorcluster)  [unwired: 9 in, 2 out]
            n723 = call "读取数据处理 (子VI).vi"("data out"=w889) -> ("系统编码ST"=→"系统编码ST":string, "命令编码CN"=w901:string, "设备编码MN"=→"设备编码MN":string, "密码PW"=→"密码PW":string, "数据"=w886:string, "拆分包及应答Flag"=→"拆分包及应答Flag":string, "时间QN"=w904:string)  [unwired: 8 in]
            "命令编码CN" <- w901
            "数据" <- w886
            "时间QN" <- w904
            n724 = Empty String/Path?(string/path=w889) -> (empty?=w898:bool)
            n725 = local read "实时小时数据上传"() -> (w897:bool)
            n726 = case shown="假" w898 {
              tunnel: w889 -> [w921 _]
              frame False {
                n727 = global write "全局1.vi" "数据输出"(w921) -> ()
                n728 = call "数据记录.vi"("写入字段"=w921) -> ("连接的字符串"=→"读取报文显示":string)  [unwired: 10 in]
                "数据输出" <- w921
              }
              frame True {
              }
            }
            n729 = local read "核查数据上传"() -> (w896:bool)
            n730 = Not(x=w897) -> (.not. x?=w895:bool)
            n731 = Not(x=w896) -> (.not. x?=w894:bool)
            n732 = And(x=w895, y=w894) -> (x .and. y?=w893:bool)
            n733 = Search/Split String(string=w904, search string/char (-)="QN=" ("搜索字符串/字符(-)")) -> (match + rest of string=w902:string)  [unwired: 1 in, 2 out]
            n734 = case shown="真" w893 {
              tunnel: w901 -> [_ w919]
              tunnel: ["" ("命令编码CN") w916] -> w899
              frame False {
              }
              frame True {
                n735 = Search/Split String(string=w919, search string/char (-)="CN=" ("搜索字符串/字符(-)")) -> (match + rest of string=w917:string)  [unwired: 1 in, 2 out]
                n736 = String Subset(string=w917, offset (0)=3 ("偏移量(0)")) -> (substring=w916:string)  [unwired: 1 in]
              }
            }
            n737 = String Subset(string=w902, offset (0)=3 ("偏移量(0)")) -> (substring=→"QN":string)  [unwired: 1 in]
            n738 = call "读取反控数据解析(子VI).vi"("数据"=w886, "命令编码CN"=w899) -> ("实时数据发送时间间隔/min"=w884:i32, "设置超时时间/min"=→"设置超时时间/min":i32)  [unwired: 8 in]
            n739 = global write "实时数据发送间隔全局.vi" "实时数据发送间隔"(w884) -> ()
            n740 = local write "实时数据发送时间间隔/min"(w884) -> ()
          }
          frame "发送数据" {
            # "table输入，选择命令编码、发送哪些数据"
            n741 = local read "table元素"() -> (w927:string)
            n742 = case shown="\"反控命令\"" w927 {
              tunnel: w926 -> [w938 w942 w944 w951]
              tunnel: [w936 w941 w945 w949] -> w923
              tunnel: [w937 w940 w946 w950] -> w925
              frame "", Default {
                n743 = global write "全局1.vi" "枚举"(w938) -> ()
                n744 = Increment(x=w938) -> (x+1=w937:i32)
                n745 = Greater Or Equal?(x=w937, y=3) -> (x >= y?=w936:bool)
              }
              frame "反控命令" {
                n746 = global write "全局 反控命令枚举.vi" "反控命令枚举"(w942) -> ()
                n747 = Increment(x=w942) -> (x+1=w940:i32)
                n748 = Greater Or Equal?(x=w940, y=2) -> (x >= y?=w941:bool)
              }
              frame "超标留样返回", "提取监测仪表时间", "提取经纬度环境信息", "提取现场系统信息" {
                n749 = global write "全局1.vi" "枚举"(w944) -> ()
                n750 = Increment(x=w944) -> (x+1=w946:i32)
                n751 = Greater Or Equal?(x=w946, y=3) -> (x >= y?=w945:bool)
              }
              frame "报警信息", "操作日志", "核查数据", "空白测试", "跨度核查", "零点核查", "实时数据", "提取集成干预", "提取加标回收", "提取平行样", "提取实时数据", "提取小时数据", "提取仪器参数", "仪器参数" {
                n752 = global read "全局 小时数据发送次数.vi" "小时数据发送次数"() -> (w953:i32)
                n753 = global read "全局 数据数组大小.vi" "数据数组大小"() -> (w948:i32)
                n754 = Greater Or Equal?(x=w953, y=w948) -> (x >= y?=w954:bool)
                n755 = case shown="真" w954 {
                  tunnel: w951 -> [w959 w966]
                  tunnel: [w959 w960] -> w955
                  frame False {
                  }
                  frame True {
                    n756 = global read "全局 小时数据发送次数.vi" "小时数据发送次数"() -> (w965:i32)
                    n757 = global read "全局 数据数组大小.vi" "数据数组大小"() -> (w962:i32)
                    n758 = Equal To 0?(x=w965) -> (x = 0?=w964:bool)
                    n759 = Equal To 0?(x=w962) -> (x = 0?=w963:bool)
                    n760 = And(x=w964, y=w963) -> (x .and. y?=w961:bool)
                    n761 = case shown="真" w961 {
                      tunnel: w966 -> [w968 _]
                      tunnel: [w967 0 ("索引")] -> w960
                      frame False {
                        n762 = Increment(x=w968) -> (x+1=w967:i32)
                      }
                      frame True {
                      }
                    }
                  }
                }
                n763 = global write "全局1.vi" "枚举"(w955) -> ()
                n764 = Equal To 0?(x=w955) -> (x = 0?=w956:bool)
                n765 = case shown="真" w956 {
                  tunnel: w955 -> [w957 _]
                  tunnel: [w957 1] -> w950
                  frame False {
                  }
                  frame True {
                  }
                }
                n766 = Greater Or Equal?(x=w950, y=2) -> (x >= y?=w949:bool)
              }
            }
            n767 = flat-sequence {
              tunnel: "table元素" -> [w981]
              tunnel: w933 -> [w980]
              tunnel: [w976] -> w932
              tunnel: [w985] -> w930
              tunnel: w932 -> [w985]
              tunnel: w931 -> [w984]
              tunnel: w923 -> [w983]
              frame #0 {
                # "数据记录"
                # "数据编码"
                n768 = local read "MN"() -> (w973:string)
                n769 = local read "QN"() -> (w979:string)
                n770 = local read "PW"() -> (w972:string)
                n771 = call "数据编码.vi"("table输入"=w981, "错误常量 2"=w980, "QN"=w979, "MN"=w973, "PW"=w972) -> ("错误常量"=w978:errorcluster, "通讯包字符串"=w977:string)  [unwired: 9 in]
                n772 = local read "数据发送通道"() -> (w975:enum16{"TCP", "VISA"})
                n773 = call "数据记录.vi"("写入字段"=w977) -> ("连接的字符串"=→"发送报文显示":string)  [unwired: 10 in]
                n774 = call "VISATCP组合选择发送.vi"("数据发送通道"=w975, "命令"="write", "error in (no error)"=w978, "写入缓冲区"=w977) -> ("错误输出"=w976:errorcluster)  [unwired: 8 in, 3 out]
              }
              frame #1 {
                n775 = case shown="假" w983 {
                  tunnel: w984 -> [w986 w998]
                  frame False {
                    n776 = Enqueue Element(queue=w986, element=T6."发送数据" ("元素")) -> ()  [unwired: 2 in, 3 out]
                  }
                  frame True {
                    n777 = local read "TCP服务端掉线计数"() -> (w993:i32)
                    n778 = Obtain Queue(name (unnamed)="重发掉线数据" ("名称（未命名）"), element data type=T12."水样测试") -> (queue out=w991:refnum<queue>, error out=w992:errorcluster)  [unwired: 3 in, 1 out]
                    n779 = Get Queue Status(queue=w991, error in (no error)=w992) -> (# elements in queue=w995:i32)  [unwired: 1 in, 7 out]
                    n780 = Not Equal To 0?(x=w995) -> (x != 0?=w996:bool)
                    n781 = Greater Or Equal?(x=w993, y=1) -> (x >= y?=w997:bool)
                    n782 = And(x=w996, y=w997) -> (x .and. y?=w989:bool)
                    n783 = case shown="真" w989 {
                      tunnel: [T6."读取数据" ("元素") T6."表格比对" ("元素")] -> w999
                      frame False {
                      }
                      frame True {
                      }
                    }
                    n784 = Enqueue Element(queue=w998, element=w999) -> ()  [unwired: 2 in, 3 out]
                  }
                }
              }
            }
            n785 = case shown="真" w923 {
              tunnel: w925 -> [w970 _]
              tunnel: [w970 1 ("索引")] -> w929
              frame False {
              }
              frame True {
              }
            }
            "查询数据发送" <- TRUE
          }
          frame "数据处理" {
            n786 = local write "空闲时间"(0.0 ("空闲时间")) -> ()
            n787 = local read "心跳包"() -> (w1010:bool)
            n788 = Equal?(x=w1008, y="实时数据") -> (x = y?=w1006:bool)
            n789 = case shown="假" w1010 {
              tunnel: w1014 -> [w1017 _]
              tunnel: w1008 -> [w1016 _]
              frame False {
                n790 = call "插入单条数据.vi"("table输入"=w1016, "插入数据"=w1017) -> ()  [unwired: 8 in, 2 out]
              }
              frame True {
              }
            }
            n791 = Select(t=0, s=w1006, f=w1004) -> (s? t:f=w1005:i32)
            n792 = Enqueue Element(queue=w1013, element=T6."表格比对" ("元素"), timeout in ms (-1)=1000 ("超时毫秒(-1)")) -> ()  [unwired: 1 in, 3 out]
          }
        }
      }
      frame Error {
        n793 = Unbundle By Name(w1021) -> ("code"=w1020:i32)
        n794 = case shown="56" w1020 {
          tunnel: w1021 -> [w1026 w1036 w1065 w1089]
          tunnel: [w1032 w1049 w1078 w1089] -> w1025
          tunnel: w1019 -> [w1033 w1044 w1073 w1086]
          frame 0, Default {
            n795 = Flush Queue(queue=w1033) -> (queue out=w1031:refnum<queue>)  [unwired: 1 in, 2 out]
            n796 = global write "全局 数据发送重叠.vi" "掉线指示灯"(TRUE ("掉线指示灯")) -> ()
            n797 = Enqueue Element(queue=w1031, element=T6."初始化" ("元素"), timeout in ms (-1)=1000 ("超时毫秒(-1)")) -> ()  [unwired: 1 in, 3 out]
            n798 = local read "数据发送通道"() -> (w1028:enum16{"TCP", "VISA"})
            n799 = call "VISATCP组合选择发送.vi"("数据发送通道"=w1028, "命令"="close", "error in (no error)"=w1026) -> ("错误输出"=w1027:errorcluster)  [unwired: 9 in, 3 out]
            n800 = call <vilib>:"Clear Errors.vi"("error in (no error)"=w1027) -> ("error out"=w1032:errorcluster)  [unwired: 5 in, 1 out]
          }
          frame 63 {
            # "TCP服务器端口掉线"
            n801 = Flush Queue(queue=w1044) -> (queue out=w1045:refnum<queue>)  [unwired: 1 in, 2 out]
            n802 = global write "全局 数据发送重叠.vi" "掉线指示灯"(TRUE ("掉线指示灯")) -> ()
            n803 = property on="TCP服务端掉线计数" class="DigNum (严格)"() -> ("Value"=w1043:i32)  [unwired: 2 in, 2 out]
            n804 = property on="TCP服务端掉线计数" class="DigNum (严格)"() -> ("Value"=w1048:i32)  [unwired: 2 in, 2 out]
            n805 = local read "数据发送通道"() -> (w1038:enum16{"TCP", "VISA"})
            n806 = Enqueue Element(queue=w1045, element=T6."初始化" ("元素"), timeout in ms (-1)=1000 ("超时毫秒(-1)")) -> ()  [unwired: 1 in, 3 out]
            n807 = Increment(x=w1048) -> (x+1=w1046:i32)
            n808 = Less Or Equal?(x=w1043, y=1) -> (x <= y?=w1041:bool)
            n809 = case shown="真" w1041 {
              frame False {
                n810 = local write "TCP掉线时间节点"("TCP掉线时间节点") -> ()
                n811 = global write "全局 数据发送重叠.vi" "TCP掉线时间节点"("TCP掉线时间节点") -> ()
              }
              frame True {
                n812 = call <vilib>:"Application Directory.vi"() -> ("Application Directory"=w1060:path)
                n813 = Build Path(base path=w1060, name or relative path="data\\Set.ini" ("名称或相对路径")) -> (appended path=w1061:path)
                n814 = Get Date/Time In Seconds() -> (seconds since 1Jan1904=w1062:timestamp)
                n815 = Format Date/Time String(time format string (%c)="%Y%m%d%H%M%S%3u" ("时间格式字符串(%c)"), seconds (now)=w1062) -> (date/time string=w1064:string)  [unwired: 1 in]
                n816 = call "格式时间字符串.vi"("字符串"=w1064) -> ("连接的字符串"=w1052:string)  [unwired: 10 in]
                n817 = call <vilib>:"Open Config Data.vi"("configuration file path"=w1061) -> ("error out"=w1057:errorcluster, "refnum"=w1058:T8)  [unwired: 8 in, 1 out]
                n818 = local write "TCP掉线时间节点"(w1052) -> ()
                n819 = call-poly <vilib>:"Write Key.vi"("section"="掉线时间存储", "error in (no error)"=w1057, "value"=w1052, "key"="掉线时间", "refnum"=w1058) -> ("error out"=w1055:errorcluster, "refnum out"=w1056:T8)  [unwired: 4 in, 1 out]
                n820 = call <vilib>:"Close Config Data.vi"("error in (no error)"=w1055, "refnum"=w1056) -> ()  [unwired: 8 in, 2 out]
              }
            }
            n821 = property on="TCP服务端掉线计数" class="DigNum (严格)"("Value"=w1046) -> ()  [unwired: 2 in, 2 out]
            n822 = call "VISATCP组合选择发送.vi"("数据发送通道"=w1038, "命令"="close", "error in (no error)"=w1036) -> ("错误输出"=w1037:errorcluster)  [unwired: 9 in, 3 out]
            n823 = call <vilib>:"Clear Errors.vi"("error in (no error)"=w1037) -> ("error out"=w1049:errorcluster)  [unwired: 5 in, 1 out]
          }
          frame 54 {
            # "TCP服务器端口掉线"
            n824 = Flush Queue(queue=w1073) -> (queue out=w1074:refnum<queue>)  [unwired: 1 in, 2 out]
            n825 = global write "全局 数据发送重叠.vi" "掉线指示灯"(TRUE ("掉线指示灯")) -> ()
            n826 = property on="TCP服务端掉线计数" class="DigNum (严格)"() -> ("Value"=w1072:i32)  [unwired: 2 in, 2 out]
            n827 = property on="TCP服务端掉线计数" class="DigNum (严格)"() -> ("Value"=w1077:i32)  [unwired: 2 in, 2 out]
            n828 = local read "数据发送通道"() -> (w1067:enum16{"TCP", "VISA"})
            n829 = Increment(x=w1077) -> (x+1=w1075:i32)
            n830 = Less Or Equal?(x=w1072, y=1) -> (x <= y?=w1070:bool)
            n831 = Enqueue Element(queue=w1074, element=T6."初始化" ("元素"), timeout in ms (-1)=1000 ("超时毫秒(-1)")) -> ()  [unwired: 1 in, 3 out]
            n832 = case shown="真" w1070 {
              frame False {
                n833 = local read "TCP掉线时间节点"() -> (w1080:string)
                n834 = local write "TCP掉线时间节点"(w1080) -> ()
                n835 = global write "全局 数据发送重叠.vi" "TCP掉线时间节点"(w1080) -> ()
              }
              frame True {
                n836 = Get Date/Time In Seconds() -> (seconds since 1Jan1904=w1082:timestamp)
                n837 = Format Date/Time String(time format string (%c)="%Y%m%d%H%M%S%3u" ("时间格式字符串(%c)"), seconds (now)=w1082) -> (date/time string=w1084:string)  [unwired: 1 in]
                n838 = call "格式时间字符串.vi"("字符串"=w1084) -> ("连接的字符串"=w1081:string)  [unwired: 10 in]
                n839 = local write "TCP掉线时间节点"(w1081) -> ()
              }
            }
            n840 = property on="TCP服务端掉线计数" class="DigNum (严格)"("Value"=w1075) -> ()  [unwired: 2 in, 2 out]
            n841 = call "VISATCP组合选择发送.vi"("数据发送通道"=w1067, "命令"="close", "error in (no error)"=w1065) -> ("错误输出"=w1066:errorcluster)  [unwired: 9 in, 3 out]
            n842 = call <vilib>:"Clear Errors.vi"("error in (no error)"=w1066) -> ("error out"=w1078:errorcluster)  [unwired: 5 in, 1 out]
          }
          frame 56 {
            n843 = Flush Queue(queue=w1086) -> (queue out=w1087:refnum<queue>)  [unwired: 1 in, 2 out]
            n844 = Enqueue Element(queue=w1087, element=T6."读取数据" ("元素"), timeout in ms (-1)=1000 ("超时毫秒(-1)")) -> ()  [unwired: 1 in, 3 out]
          }
        }
        n845 = call <vilib>:"Clear Errors.vi"("error in (no error)"=w1025) -> ("error out"=w1024:errorcluster)  [unwired: 5 in, 1 out]
      }
    }
    n846 = Wait (ms)(milliseconds to wait=u32 300 ("等待时间（毫秒）")) -> ()  [unwired: 1 out]
  }
  n847 = flat-sequence {
    frame #0 {
      w1105 = "线程一自主部署站点保存"
      (unwired) path "C:/LabVIEW Project/builds/平台数据发送系统" ("Application Directory")
      w1167 = "" ("参数")
      w1092 = FALSE ("数据发送中断")
      w1138 = 0 ("数值")
      # "版本改动:增加了远程反控命令，和仪器端双向通讯，modbus TCP读写"
      # "ST参数选择"
      n848 = property class="VI"() -> ("Panel"=w1171:refnum<vi>)  [unwired: 2 in, 2 out]
      n849 = global write "全局 实时数据参数.vi" "参数"(w1167) -> ()
      n850 = local write "核查数据上传"(w1092) -> ()
      n851 = local write "查询数据发送"(w1092) -> ()
      n852 = local write "心跳包"(w1092) -> ()
      n853 = global write "全局 小时数据发送次数.vi" "小时数据发送次数"(w1138) -> ()
      n854 = local write "实时小时数据上传"(w1092) -> ()
      n855 = local write "系统状态改变"(w1092) -> ()
      n856 = property class="Pnl"(reference=w1171) -> ("Panes[]"=w1170:refnum<vi>[])  [unwired: 1 in, 2 out]
      n857 = global write "全局 实时数据参数.vi" "data"(string[][] [] ("data")) -> ()
      n858 = property on="窗格" class="Pane"("Origin"=T11 {"Horizontal"=0, "Vertical"=0} ("原点")) -> ()  [unwired: 2 in, 2 out]
      n859 = local write "空闲时间"(0.0 ("try")) -> ()
      n860 = global write "全局1.vi" "枚举"(enum16{"返回请求应答", "上传数据", "返回执行结果"}."返回请求应答" ("枚举")) -> ()
      n861 = global write "全局 实时数据参数.vi" "连接的字符串"(w1167) -> ()
      n862 = call <vilib>:"Application Directory.vi"() -> ("Application Directory"=w1165:path)
      n863 = for {
        tunnel: w1170 -> [w1182] mode=indexing
        tunnel: u32 15592941 ("窗格颜色") -> [w1183]
        n864 = property class="Pane"(reference=w1182, "PaneColor"=w1183) -> ()  [unwired: 1 in, 2 out]
      }
      n865 = Build Path(base path=w1165, name or relative path="data\\Set.ini" ("名称或相对路径")) -> (appended path=w1163:path)
      n866 = call <vilib>:"Open Config Data.vi"("configuration file path"=w1163) -> ("error out"=w1161:errorcluster, "refnum"=w1162:T8)  [unwired: 8 in, 1 out]
      n867 = call <vilib>:"Application Directory.vi"() -> ("Application Directory"=w1128:path)
      n868 = call-poly <vilib>:"Read Key.vi"("section"=w1105, "error in (no error)"=w1161, "key"="站点名称", "refnum"=w1162) -> ("error out"=w1158:errorcluster, "value"=w1119:string, "refnum out"=w1159:T8)  [unwired: 4 in, 1 out]
      n869 = call <vilib>:"Application Directory.vi"() -> ("Application Directory"=w1096:path)
      n870 = call <vilib>:"Application Directory.vi"() -> ("Application Directory"=w1124:path)
      n871 = call <vilib>:"Recursive File List.vi"("pattern"="*.exe", "Folder Path"=w1128) -> ("All Files in Dir"=w1136:path[])  [unwired: 5 in, 4 out]
      n872 = Build Path(base path=w1096, name or relative path="data\\sys.ini" ("名称或相对路径")) -> (appended path=w1094:path)
      n873 = local write "站点名称"(w1119) -> ()
      n874 = Build Path(base path=w1124, name or relative path="data\\background.jpg" ("名称或相对路径")) -> (appended path=w1123:path)
      n875 = call <vilib>:"Open Config Data.vi"("configuration file path"=w1094) -> ("error out"=w1100:errorcluster, "refnum"=w1099:T8)  [unwired: 8 in, 1 out]
      n876 = Index Array(array=w1136) -> (element=w1135:path)  [unwired: 1 in]
      n877 = Get Date/Time In Seconds() -> (seconds since 1Jan1904=w1175:timestamp)
      n878 = call <vilib>:"Read JPEG File.vi"("path to JPEG file"=w1123) -> ("error out"=w1121:errorcluster, "image data"=w1122:T13)  [unwired: 8 in, 1 out]
      n879 = vi-ref "断电保存全局.vi"() -> (w1098:refnum<vi>)
      n880 = Format Date/Time String(time format string (%c)="%Y%m%d%H%M%S%3u" ("时间格式字符串(%c)"), seconds (now)=w1175) -> (date/time string=w1174:string)  [unwired: 1 in]
      n881 = call-poly <vilib>:"Read Key.vi"("section"=w1105, "error in (no error)"=w1158, "key"="站点设备", "refnum"=w1159) -> ("error out"=w1155:errorcluster, "value"=w1118:string, "refnum out"=w1156:T8)  [unwired: 4 in, 1 out]
      n882 = File/Directory Info(path=w1135) -> (last mod=w1134:timestamp)  [unwired: 1 in, 6 out]
      n883 = call <vilib>:"FileVersionInfo.vi"("Application Path in"=w1135) -> ("error out"=w1120:errorcluster, "File Version Info"=w1131:string)  [unwired: 7 in, 2 out]
      n884 = call <userlib>:"Read Panel from INI__ogtk.vi"("error in (no error)"=w1100, "VI ref"=w1098, "refnum"=w1099) -> ("error out"=w1093:errorcluster, "refnum out"=w1097:T8)  [unwired: 7 in]
      n885 = property on="窗格" class="Pane"("BackgroundImage"=w1122) -> ()  [unwired: 2 in, 2 out]
      n886 = Search and Replace String(input string=w1174, search string="." ("搜索字符串")) -> (result string=w1172:string)  [unwired: 6 in, 3 out]
      n887 = Format Date/Time String(time format string (%c)="\n%Y%m%d%H%M" ("时间格式字符串(%c)"), seconds (now)=w1134) -> (date/time string=w1130:string)  [unwired: 1 in]
      n888 = local write "站点设备"(w1118) -> ()
      n889 = case shown="错误" w1093 {
        frame No Error {
        }
        frame Error {
          n890 = global write "断电保存全局.vi" "数据发送协议"(enum16{"2005-212协议", "2017-212协议"}."2017-212协议" ("数据发送协议")) -> ()
          n891 = global write "断电保存全局.vi" "判断数据反馈"(TRUE ("判断数据反馈")) -> ()
          n892 = global write "断电保存全局.vi" "数据发送通道"(enum16{"TCP", "VISA"}."TCP" ("数据发送通道")) -> ()
        }
      }
      n893 = call <vilib>:"Close Config Data.vi"("error in (no error)"=w1093, "refnum"=w1097) -> ()  [unwired: 8 in, 2 out]
      n894 = call-poly <vilib>:"Read Key.vi"("section"=w1105, "error in (no error)"=w1155, "key"="IP", "refnum"=w1156) -> ("error out"=w1152:errorcluster, "value"=w1117:string, "refnum out"=w1153:T8)  [unwired: 4 in, 1 out]
      n895 = Concatenate Strings("V" ("字符串"), w1131, w1130) -> (→"软件版本":string)
      n896 = local write "QN"(w1172) -> ()
      n897 = call <vilib>:"Simple Error Handler.vi"("error in (no error)"=w1120) -> ()  [unwired: 4 in, 5 out]
      n898 = call <vilib>:"Simple Error Handler.vi"("error in (no error)"=w1121) -> ()  [unwired: 4 in, 5 out]
      n899 = local write "IP"(w1117) -> ()
      n900 = call-poly <vilib>:"Read Key.vi"("section"=w1105, "error in (no error)"=w1152, "key"="PORT", "refnum"=w1153) -> ("error out"=w1148:errorcluster, "value"=w1116:string, "refnum out"=w1149:T8)  [unwired: 4 in, 1 out]
      n901 = call <vilib>:"Application Directory.vi"() -> ("Application Directory"=w1127:path)
      n902 = local write "PORT"(w1116) -> ()
      n903 = call "查询启动项.vi"("启动文件路径"=w1127) -> ("包含启动项"=w1126:bool)  [unwired: 9 in, 1 out]
      n904 = call-poly <vilib>:"Read Key.vi"("section"=w1105, "error in (no error)"=w1148, "key"="MN", "refnum"=w1149) -> ("error out"=w1112:errorcluster, "value"=w1115:string, "refnum out"=w1113:T8)  [unwired: 4 in, 1 out]
      n905 = local write "MN"(w1115) -> ()
      n906 = local write "开机启动"(w1126) -> ()
      n907 = call-poly <vilib>:"Read Key.vi"("section"=w1105, "error in (no error)"=w1112, "key"="PW", "refnum"=w1113) -> ("error out"=w1110:errorcluster, "value"=w1114:string, "refnum out"=w1111:T8)  [unwired: 4 in, 1 out]
      n908 = local write "PW"(w1114) -> ()
      n909 = call-poly <vilib>:"Read Key.vi"("section"=w1105, "error in (no error)"=w1110, "key"="VISA", "refnum"=w1111) -> ("error out"=w1106:errorcluster, "value"=w1108:string, "refnum out"=w1107:T8)  [unwired: 4 in, 1 out]
      n910 = local write "VISA resource name"(w1108) -> ()
      n911 = call-poly <vilib>:"Read Key.vi"("section"=w1105, "error in (no error)"=w1106, "key"="BAUDRATE", "refnum"=w1107) -> ("error out"=w1101:errorcluster, "value"=w1103:i32, "refnum out"=w1102:T8)  [unwired: 4 in, 1 out]
      n912 = local write "baud rate"(w1103) -> ()
      n913 = call-poly <vilib>:"Read Key.vi"("section"="系统编码选择", "error in (no error)"=w1101, "key"="系统编码", "refnum"=w1102) -> ("error out"=w1142:errorcluster, "value"=w1144:string, "refnum out"=w1143:T8)  [unwired: 4 in, 1 out]
      n914 = local write "系统编码选择框"(w1144) -> ()
      n915 = call-poly <vilib>:"Read Key.vi"("section"="掉线时间存储", "error in (no error)"=w1142, "key"="掉线时间", "refnum"=w1143) -> ("error out"=w1090:errorcluster, "value"=w1139:string, "refnum out"=w1091:T8)  [unwired: 4 in, 1 out]
      n916 = global write "全局 数据发送重叠.vi" "TCP掉线时间节点"(w1139) -> ()
      n917 = local write "TCP掉线时间节点"(w1139) -> ()
      n918 = call <vilib>:"Close Config Data.vi"("error in (no error)"=w1090, "refnum"=w1091) -> ()  [unwired: 8 in, 2 out]
      "TCP服务端掉线计数" <- w1138
    }
  }
  n919 = vi-ref "数据传输系统.lvlib:最小窗口后台运行(子VI).vi"() -> (w39:refnum<vi>)
  n920 = property class="VI"(reference=w39) -> ("Name"=w40:string)  [unwired: 1 in, 2 out]
  n921 = Open VI Reference(type specifier VI Refnum (for type only)=refnum<vi> refnum, vi path=w40, options=128 ("选项")) -> (vi reference=w42:refnum<vi>, error out=w44:errorcluster)  [unwired: 3 in]
  n922 = call-by-ref "?"(reference=w42, error in=w44) -> (reference out=w46:refnum<vi>, error out=w45:errorcluster)  [unwired: 11 in, 1 out]
  n923 = Close Reference(reference=w46, error in (no error)=w45) -> ()  [unwired: 1 out]
